vi "ADC Config Panel.vi"(8 "error in":errorcluster, 11 "adc session in":T2={"niScope"={"channel cfg"=[], "sessions"=[], "multi cards"=FALSE, "channels"=0, "type"=enum."n/a", "memory [B/chn]"=0, "ext. clock [Hz]"=0.0, "samples count"=0, "use streaming"=FALSE, "proc setup"={"packet size [smpl]"=0, "current timeout [s]"=0.0, "blk2blk timeout [s]"=0.0, "event time"=timestamp(0 s since 1904-01-01), "temp sampl T [s]"=0.0, "data queue"=refnum, "stop notifier"=refnum, "proc ref"=refnum}, "sample width [B]"=0, "ranges [V]"=[], "trigger setup"={"coupling"=1, "level [V]"=0.0, "slope"=0, "mode"=enum."Immediate", "pre-trigger [%]"=0.0}, "fs [Hz]"=0.0, "bitres [bit]"=0, "clock source"=enum."VAL_NO_SOURCE"}, "3458A"={"channels"=[], "sync unit"={"VISA"="", "type"=enum."Picotest U6200A"}, "awg unit"={"type"=enum."Agilent 331xxA to 332xxA", "VISA"="", "enable 10MHz ref"=FALSE, "cmi ckd2"={"VISA"="", "clock source"=enum."Auto", "manual ref clk"=FALSE, "ref clock [Hz]"=0.0, "div mode"=enum."Set divisor directly"}, "cmi sync v3"={"VISA"="", "baud rate [bd/s]"=115200, "source"=enum."Auto", "hv range"=enum."1kV", "fsrc is fixed"=FALSE, "fsrc [Hz]"=10000000.0, "freq integ [s]"=1.0, "freq filter"=5, "trig level"=enum."TTL 5V", "chn1 mode"=enum."Source divider", "chn1 level"=enum."Positive 5V", "chn2 mode"=enum."Source divider", "chn2 level"=enum."Positive 5V", "chn2 div"=1, "chn3 mode"=enum."Chn 1 Active", "chn3 level"=enum."Positive 5V", "chn1 div entry"=enum."Calculate nearest divisor from measured fx", "chn1 dev limit [%]"=1.0, "chn1 check dev"=FALSE}, "trigger"={"source"=enum."Immediate", "slope"=enum."POS", "coupling"=enum."DC", "level [V]"=0.0, "hysteresis [V]"=0.0, "pre-trigger [%]"=0.0}, "HMF2500 cfg"={"Baud Rate"=9600, "Parity"=0, "Data Bits"=8, "Flow Control"=4}}, "sync mode"=enum."MASTER-SLAVE, MASTER clocked by TIMER", "streaming mode"=FALSE, "idn mode"=enum."Auto", "sampling mode"=enum."DCV", "sample memory [B]"=0, "proc setup"={"channel id"=0, "packet size [smpl]"=0, "current timeout [s]"=0.0, "blk2blk timeout [s]"=0.0, "event time"=timestamp(0 s since 1904-01-01), "stop notifier"=refnum, "data queues"=[], "proc refs"=[], "bus semaphore"=refnum}, "sample size [B]"=0, "sample count"=0, "aux data"={"channel id"=0, "valid?"=[], "gain [V]"=[], "timestamp [s]"=[], "Ts [s]"=0.0, "abs timestamp"=timestamp(0 s since 1904-01-01), "t [deg C]"=[], "multiplex timestamp [s]"=-1.0, "only multiplex?"=FALSE, "multiplex smpl offset"=0, "overflow?"=FALSE}, "ranges [V]"=[], "aperture [s]"=0.0, "LEVEL trigger"={"edge"=enum."POS", "level [V]"=0.0, "coupling"=enum."DC"}, "trigger mode"=enum."AUTO", "measure temp.?"=FALSE, "disp mesages"=[], "shared bus?"=FALSE, "disable display?"=FALSE, "aper mode"=enum."Manual", "aper rules"=[], "multiplex"={"cycles"=0, "delay [s]"=0.0, "enabled"=FALSE, "overhead [s]"=1.0, "tot smpls"=0, "sub-rec"=0, "overhead [%]"=0.0, "emulated"=FALSE}, "F8588 lpf"=enum."Off", "F8588 pll"=enum."Off", "F8588 couple"=enum."DC, auto", "fs"={"freq mode"=enum."fs or Ts", "fs [Hz]"=0.0, "fref [Hz]"=0.0, "mul"=0.0, "div"=0.0}, "fs mode"=enum."fs or Ts"}, "dsdll"={"dsdll"={"dsdll path"=path "", "dsdll handle"=[], "output devices"=[], "capture devices"=[]}, "channels"=0, "device id"=0, "channel idns"=[], "proc setup"={"packet size [smpl]"=0, "current timeout [s]"=0.0, "blk2blk timeout [s]"=0.0, "event time"=timestamp(0 s since 1904-01-01), "data queue"=refnum, "stop notifier"=refnum, "proc ref"=refnum}, "samples count"=0, "fs [Hz]"=0.0}, "type"=enum."niScope", "channel idn str"=[], "aux instr idn str"=[], "modified?"=FALSE, "simadc"={"channels"=[], "range [V]"=0.0, "Ts step [s]"=0.0, "time [s]"=0.0, "fs [Hz]"=0.0, "count"=0, "smpl offset"=0, "set count"=0, "bit res"=0}, "force rst?"=FALSE, "exit mode"=enum."Immediate reset", "exit dly"=0.0, "exit tmr"=timestamp(0 s since 1904-01-01), "busy?"=FALSE, "accessed?"=FALSE, "multiplex"={"Type"=enum."Dummy", "gen com ssn"={"visa"="", "primary"=enum."None", "secondary"=enum."None", "channels"=[]}, "delay before [s]"=0.0, "delay post [s]"=0.0, "sequence"=[], "enabled"=FALSE, "ref timestamp [s]"=0.0, "idn string"="", "dev niScope"="", "niScope idx"=0, "QPMX ssn"={"visa"="", "switch mode"=enum."Switched by TWM", "sequence"=[], "timing delays"=[], "polarity"=enum."Positive", "ss delay (s)"=2.0, "internal timer (s)"=1.0, "Last loaded sequence file"=path "", "startup delay (s)"=2.0}, "VISA mux ssn"={"VISA"="", "paths"=[], "idn command"="", "serial cfg"={"Baud rate"=9600, "Data bits"=8, "Parity"=0, "Stop bits"=10, "Flow control"=0, "End Mode Read"=enum."None", "End Mode Write"=enum."None", "Term character"=0, "Term enable"=FALSE}}}, "keysight dso"={"VISA"="", "channels"=[], "bw limit [Hz]"=0.0, "resolution"=enum."Basic", "trig noise reject"=enum."Normal", "N"=0, "trigger config"={"trigger source"=enum."Immediate", "trigger slope"=enum."Negative", "level [V]"=0.0, "hysteresis [V]"=0.001, "pre-trig [%]"=50}, "fs [Hz]"=0.0, "timeout stop"=timestamp(0 s since 1904-01-01), "waiting for opc"=FALSE, "fetch offset [smpl]"=0, "abs timestamp"=timestamp(0 s since 1904-01-01), "ranges [V]"=[], "decimation"=0.0, "ext ref"=FALSE}, "cdaq"={"mclk [Hz]"=12800000.0, "ADC task"="", "mclk reference"="", "fs [Hz]"=50000.0, "queue adc cmd"=refnum, "queue adc data"=refnum, "adc proc ref"=refnum, "channels"=[], "last channels"=[], "timeout"=timestamp(0 s since 1904-01-01), "N"=1000, "mclk mode"=enum."Free running", "ext mclk source"=""}, "ignore overload"=FALSE} {"cdaq"."last channels"."Channel id" min=0 step=1; "cdaq"."channels"."Channel id" min=0 step=1; "keysight dso"."bw limit [Hz]" format="%#_6p"; "keysight dso"."channels"."Offset [V]" format="%#_6p"; "keysight dso"."channels"."Range [Vpk]" min=0.0 format="%#_6p"; "keysight dso"."channels"."Channel" min=1; "multiplex"."VISA mux ssn"."serial cfg"."Flow control" items=["None", "XON/XOFF", "CTS/RTS", "XON/XOFF + CTS/RTS", "DTR/DSR", "XON/XOFF + DTR/DSR"]; "multiplex"."VISA mux ssn"."serial cfg"."Stop bits" items=["1 bit"=10, "1.5 bits"=15, "2 bits"=20]; "multiplex"."VISA mux ssn"."serial cfg"."Parity" items=["None", "Odd", "Even", "Mark", "Space"]; "multiplex"."VISA mux ssn"."serial cfg"."Data bits" items=["5 bits"=5, "6 bits"=6, "7 bits"=7, "8 bits"=8]; "multiplex"."VISA mux ssn"."serial cfg"."Baud rate" items=["150 Bd"=150, "300 Bd"=300, "600 Bd"=600, "1200 Bd"=1200, "2400 Bd"=2400, "4800 Bd"=4800, "9600 Bd"=9600, "19.2 kBd"=19200, "38.4 kBd"=38400, "57.6 kBd"=57600, "115.2 kBd"=115200]; "multiplex"."QPMX ssn"."startup delay (s)" min=0.0 step=1.0; "multiplex"."QPMX ssn"."internal timer (s)" min=0.0 step=1.0; "multiplex"."QPMX ssn"."ss delay (s)" min=0.0 step=1.0; "multiplex"."QPMX ssn"."timing delays" min=1 max=255 step=1; "3458A"."awg unit"."HMF2500 cfg"."Flow Control" items=["None", "XON/XOFF", "RTS/CTS", "XON/XOFF & RTS/CTS", "DTR/DSR", "XON/XOFF & DTR/DSR"]; "3458A"."awg unit"."HMF2500 cfg"."Data Bits" items=["7"=7, "8"=8]; "3458A"."awg unit"."HMF2500 cfg"."Parity" items=["None", "Odd", "Even", "Mark", "Space"]; "3458A"."awg unit"."HMF2500 cfg"."Baud Rate" items=["300"=300, "600"=600, "1200"=1200, "2400"=2400, "4800"=4800, "9600"=9600, "19200"=19200]; "3458A"."awg unit"."cmi sync v3"."chn2 div" min=1 max=100000000 step=1; "3458A"."awg unit"."cmi sync v3"."fsrc [Hz]" format="%_8p"; "3458A"."channels"."Range [Vpk]" min=0.0; "niScope"."trigger setup"."pre-trigger [%]" format="%.2f"; "niScope"."trigger setup"."level [V]" format="%.2f"; "niScope"."trigger setup"."coupling" items=["AC"=0, "DC"=1, "HF Reject"=3, "LF Reject"=4, "AC Plus HF Reject"=1001]; "niScope"."channel cfg"."Range [Vpk]" min=0.0; "niScope"."channel cfg"."Channel" min=0}) -> (0 "error out":errorcluster, 3 "adc session out":T2={"niScope"={"channel cfg"=[], "sessions"=[], "multi cards"=FALSE, "channels"=0, "type"=enum."n/a", "memory [B/chn]"=0, "ext. clock [Hz]"=0.0, "samples count"=0, "use streaming"=FALSE, "proc setup"={"packet size [smpl]"=0, "current timeout [s]"=0.0, "blk2blk timeout [s]"=0.0, "event time"=timestamp(0 s since 1904-01-01), "temp sampl T [s]"=0.0, "data queue"=refnum, "stop notifier"=refnum, "proc ref"=refnum}, "sample width [B]"=0, "ranges [V]"=[], "trigger setup"={"coupling"=1, "level [V]"=0.0, "slope"=0, "mode"=enum."Immediate", "pre-trigger [%]"=0.0}, "fs [Hz]"=0.0, "bitres [bit]"=0, "clock source"=enum."VAL_NO_SOURCE"}, "3458A"={"channels"=[], "sync unit"={"VISA"="", "type"=enum."Picotest U6200A"}, "awg unit"={"type"=enum."Agilent 331xxA to 332xxA", "VISA"="", "enable 10MHz ref"=FALSE, "cmi ckd2"={"VISA"="", "clock source"=enum."Auto", "manual ref clk"=FALSE, "ref clock [Hz]"=0.0, "div mode"=enum."Set divisor directly"}, "cmi sync v3"={"VISA"="", "baud rate [bd/s]"=115200, "source"=enum."Auto", "hv range"=enum."1kV", "fsrc is fixed"=FALSE, "fsrc [Hz]"=10000000.0, "freq integ [s]"=1.0, "freq filter"=5, "trig level"=enum."TTL 5V", "chn1 mode"=enum."Source divider", "chn1 level"=enum."Positive 5V", "chn2 mode"=enum."Source divider", "chn2 level"=enum."Positive 5V", "chn2 div"=1, "chn3 mode"=enum."Chn 1 Active", "chn3 level"=enum."Positive 5V", "chn1 div entry"=enum."Calculate nearest divisor from measured fx", "chn1 dev limit [%]"=1.0, "chn1 check dev"=FALSE}, "trigger"={"source"=enum."Immediate", "slope"=enum."POS", "coupling"=enum."DC", "level [V]"=0.0, "hysteresis [V]"=0.0, "pre-trigger [%]"=0.0}, "HMF2500 cfg"={"Baud Rate"=9600, "Parity"=0, "Data Bits"=8, "Flow Control"=4}}, "sync mode"=enum."MASTER-SLAVE, MASTER clocked by TIMER", "streaming mode"=FALSE, "idn mode"=enum."Auto", "sampling mode"=enum."DCV", "sample memory [B]"=0, "proc setup"={"channel id"=0, "packet size [smpl]"=0, "current timeout [s]"=0.0, "blk2blk timeout [s]"=0.0, "event time"=timestamp(0 s since 1904-01-01), "stop notifier"=refnum, "data queues"=[], "proc refs"=[], "bus semaphore"=refnum}, "sample size [B]"=0, "sample count"=0, "aux data"={"channel id"=0, "valid?"=[], "gain [V]"=[], "timestamp [s]"=[], "Ts [s]"=0.0, "abs timestamp"=timestamp(0 s since 1904-01-01), "t [deg C]"=[], "multiplex timestamp [s]"=-1.0, "only multiplex?"=FALSE, "multiplex smpl offset"=0, "overflow?"=FALSE}, "ranges [V]"=[], "aperture [s]"=0.0, "LEVEL trigger"={"edge"=enum."POS", "level [V]"=0.0, "coupling"=enum."DC"}, "trigger mode"=enum."AUTO", "measure temp.?"=FALSE, "disp mesages"=[], "shared bus?"=FALSE, "disable display?"=FALSE, "aper mode"=enum."Manual", "aper rules"=[], "multiplex"={"cycles"=0, "delay [s]"=0.0, "enabled"=FALSE, "overhead [s]"=1.0, "tot smpls"=0, "sub-rec"=0, "overhead [%]"=0.0, "emulated"=FALSE}, "F8588 lpf"=enum."Off", "F8588 pll"=enum."Off", "F8588 couple"=enum."DC, auto", "fs"={"freq mode"=enum."fs or Ts", "fs [Hz]"=0.0, "fref [Hz]"=0.0, "mul"=0.0, "div"=0.0}, "fs mode"=enum."fs or Ts"}, "dsdll"={"dsdll"={"dsdll path"=path "", "dsdll handle"=[], "output devices"=[], "capture devices"=[]}, "channels"=0, "device id"=0, "channel idns"=[], "proc setup"={"packet size [smpl]"=0, "current timeout [s]"=0.0, "blk2blk timeout [s]"=0.0, "event time"=timestamp(0 s since 1904-01-01), "data queue"=refnum, "stop notifier"=refnum, "proc ref"=refnum}, "samples count"=0, "fs [Hz]"=0.0}, "type"=enum."niScope", "channel idn str"=[], "aux instr idn str"=[], "modified?"=FALSE, "simadc"={"channels"=[], "range [V]"=0.0, "Ts step [s]"=0.0, "time [s]"=0.0, "fs [Hz]"=0.0, "count"=0, "smpl offset"=0, "set count"=0, "bit res"=0}, "force rst?"=FALSE, "exit mode"=enum."Immediate reset", "exit dly"=0.0, "exit tmr"=timestamp(0 s since 1904-01-01), "busy?"=FALSE, "accessed?"=FALSE, "multiplex"={"Type"=enum."Dummy", "gen com ssn"={"visa"="", "primary"=enum."None", "secondary"=enum."None", "channels"=[]}, "delay before [s]"=0.0, "delay post [s]"=0.0, "sequence"=[], "enabled"=FALSE, "ref timestamp [s]"=0.0, "idn string"="", "dev niScope"="", "niScope idx"=0, "QPMX ssn"={"visa"="", "switch mode"=enum."Switched by TWM", "sequence"=[], "timing delays"=[], "polarity"=enum."Positive", "ss delay (s)"=2.0, "internal timer (s)"=1.0, "Last loaded sequence file"=path "", "startup delay (s)"=2.0}, "VISA mux ssn"={"VISA"="", "paths"=[], "idn command"="", "serial cfg"={"Baud rate"=9600, "Data bits"=8, "Parity"=0, "Stop bits"=10, "Flow control"=0, "End Mode Read"=enum."None", "End Mode Write"=enum."None", "Term character"=0, "Term enable"=FALSE}}}, "keysight dso"={"VISA"="", "channels"=[], "bw limit [Hz]"=0.0, "resolution"=enum."Basic", "trig noise reject"=enum."Normal", "N"=0, "trigger config"={"trigger source"=enum."Immediate", "trigger slope"=enum."Negative", "level [V]"=0.0, "hysteresis [V]"=0.001, "pre-trig [%]"=50}, "fs [Hz]"=0.0, "timeout stop"=timestamp(0 s since 1904-01-01), "waiting for opc"=FALSE, "fetch offset [smpl]"=0, "abs timestamp"=timestamp(0 s since 1904-01-01), "ranges [V]"=[], "decimation"=0.0, "ext ref"=FALSE}, "cdaq"={"mclk [Hz]"=12800000.0, "ADC task"="", "mclk reference"="", "fs [Hz]"=50000.0, "queue adc cmd"=refnum, "queue adc data"=refnum, "adc proc ref"=refnum, "channels"=[], "last channels"=[], "timeout"=timestamp(0 s since 1904-01-01), "N"=1000, "mclk mode"=enum."Free running", "ext mclk source"=""}, "ignore overload"=FALSE} {"cdaq"."last channels"."Channel id" min=0 step=1; "cdaq"."channels"."Channel id" min=0 step=1; "keysight dso"."bw limit [Hz]" format="%#_6p"; "keysight dso"."channels"."Offset [V]" format="%#_6p"; "keysight dso"."channels"."Range [Vpk]" min=0.0 format="%#_6p"; "keysight dso"."channels"."Channel" min=1; "multiplex"."VISA mux ssn"."serial cfg"."Flow control" items=["None", "XON/XOFF", "CTS/RTS", "XON/XOFF + CTS/RTS", "DTR/DSR", "XON/XOFF + DTR/DSR"]; "multiplex"."VISA mux ssn"."serial cfg"."Stop bits" items=["1 bit"=10, "1.5 bits"=15, "2 bits"=20]; "multiplex"."VISA mux ssn"."serial cfg"."Parity" items=["None", "Odd", "Even", "Mark", "Space"]; "multiplex"."VISA mux ssn"."serial cfg"."Data bits" items=["5 bits"=5, "6 bits"=6, "7 bits"=7, "8 bits"=8]; "multiplex"."VISA mux ssn"."serial cfg"."Baud rate" items=["150 Bd"=150, "300 Bd"=300, "600 Bd"=600, "1200 Bd"=1200, "2400 Bd"=2400, "4800 Bd"=4800, "9600 Bd"=9600, "19.2 kBd"=19200, "38.4 kBd"=38400, "57.6 kBd"=57600, "115.2 kBd"=115200]; "multiplex"."QPMX ssn"."startup delay (s)" min=0.0 step=1.0; "multiplex"."QPMX ssn"."internal timer (s)" min=0.0 step=1.0; "multiplex"."QPMX ssn"."ss delay (s)" min=0.0 step=1.0; "multiplex"."QPMX ssn"."timing delays" min=1 max=255 step=1; "3458A"."awg unit"."HMF2500 cfg"."Flow Control" items=["None", "XON/XOFF", "RTS/CTS", "XON/XOFF & RTS/CTS", "DTR/DSR", "XON/XOFF & DTR/DSR"]; "3458A"."awg unit"."HMF2500 cfg"."Data Bits" items=["7"=7, "8"=8]; "3458A"."awg unit"."HMF2500 cfg"."Parity" items=["None", "Odd", "Even", "Mark", "Space"]; "3458A"."awg unit"."HMF2500 cfg"."Baud Rate" items=["300"=300, "600"=600, "1200"=1200, "2400"=2400, "4800"=4800, "9600"=9600, "19200"=19200]; "3458A"."awg unit"."cmi sync v3"."chn2 div" min=1 max=100000000 step=1; "3458A"."awg unit"."cmi sync v3"."fsrc [Hz]" format="%_8p"; "3458A"."channels"."Range [Vpk]" min=0.0; "niScope"."trigger setup"."pre-trigger [%]" format="%.2f"; "niScope"."trigger setup"."level [V]" format="%.2f"; "niScope"."trigger setup"."coupling" items=["AC"=0, "DC"=1, "HF Reject"=3, "LF Reject"=4, "AC Plus HF Reject"=1001]; "niScope"."channel cfg"."Range [Vpk]" min=0.0; "niScope"."channel cfg"."Channel" min=0})   [LabVIEW 2020]
doc: "Configuration panel for digitizer."
uses:
  drivers/niScope/niScope Virtual Channel Config.ctl
  drivers/niScope/niScope Virtual Channel Mode.ctl
  drivers/niScope/niScope Virtual Channel Input Z.ctl
  drivers/niScope/niScope Virtual Channel Coupling.ctl
  ADC Type.ctl
  drivers/DMM/3458A Virtual Channel Config.ctl
  drivers/AWG/AWG Type.ctl
  drivers/DMM/3458A Idn Mode.ctl
  drivers/Counter/Counter Type.ctl
  drivers/DMM/3458A Digitizing Low Levels/Configure/Sampling Mode.ctl
  drivers/DMM/3458A Sync Mode.ctl
  ADC Session.ctl
  drivers/niScope/niScope Session.ctl
  drivers/niScope/niScope Type.ctl
  drivers/niScope/niScope Digitizing Process Options.ctl
  drivers/niScope/niScope Data Packet.ctl
  drivers/niScope/niScope Trigger Setup.ctl
  <instrlib>/niScope/Controls/niScope trigger coupling.ctl
  <instrlib>/niScope/Controls/niScope trigger slope.ctl
  drivers/niScope/niScope Reference Clock.ctl
  drivers/DMM/3458A Digitizer Session.ctl
  drivers/Counter/Counter Session.ctl
  drivers/AWG/AWG Session.ctl
  drivers/AWG/CMI Clock Divider v2/CMI ckd2 Session.ctl
  drivers/AWG/CMI Clock Divider v2/CMI ckd2 Source Mode.ctl
  drivers/AWG/CMI Clock Divider v2/CMI ckd2 Divisor Mode.ctl
  drivers/AWG/CMI Sync V3/CMI Sync V3 session.ctl
  drivers/AWG/CMI Sync V3/Configure/CMI Sync V3 Reference Clock Source.ctl
  drivers/AWG/CMI Sync V3/Configure/CMI Sync V3 HV input Range.ctl
  drivers/AWG/CMI Sync V3/Configure/CMI Sync V3 Trigger Input Level.ctl
  drivers/AWG/CMI Sync V3/Configure/CMI Sync V3 Channel 1 Mode.ctl
  drivers/AWG/CMI Sync V3/Configure/CMI Sync V3 Channel Output Levels.ctl
  drivers/AWG/CMI Sync V3/Configure/CMI Sync V3 Channel 2 Mode.ctl
  drivers/AWG/CMI Sync V3/Configure/CMI Sync V3 Channel 3 Mode.ctl
  drivers/AWG/CMI Sync V3/Configure/CMI Sync V3 Channel 1 Divisor Entry Mode.ctl
  ADC Trig Config.ctl
  ADC Trig Mode Source.ctl
  ADC Trig Slope.ctl
  ADC Trig Coupling.ctl
  drivers/AWG/RaS HMF2500/HMF2500 Config.ctl
  drivers/DMM/3458A Digitizing Process Options.ctl
  drivers/DMM/3458A Data Packet.ctl
  drivers/DMM/3458A Aux Record Data.ctl
  drivers/DMM/3458A Digitizing Low Levels/Configure/Level Setup.ctl
  drivers/DMM/3458A Digitizing Low Levels/Configure/First Sample Trigger.ctl
  drivers/DMM/3458A Aperture Selection Mode.ctl
  drivers/DMM/3458A Multiplexing Config.ctl
  drivers/Fluke 8588A/F8588A Low Pass Filter.ctl
  drivers/Fluke 8588A/F8588A Phase Lock.ctl
  drivers/Fluke 8588A/F8588A Coupling.ctl
  drivers/DMM/3458A Sampling Rate.ctl
  drivers/AWG/AWG Clock Setup Mode.ctl
  drivers/DMM/3458A Sample Rate Mode.ctl
  drivers/dsdll/DSDLL Session.ctl
  drivers/dsdll/dsdll/dsdll_instance.ctl
  drivers/dsdll/dsdll/dsdll_device_record.ctl
  drivers/dsdll/DSDLL Process Config.ctl
  drivers/dsdll/DSDLL Data Packet.ctl
  drivers/simulated_adc/SimAdc Config.ctl
  drivers/simulated_adc/SimAdc Channel Cfg.ctl
  ADC On Close Action.ctl
  Multiplexer/MPX Session.ctl
  Multiplexer/MPX Type.ctl
  drivers/Multiplexers/Generic COM/GCOMM Session.ctl
  drivers/Multiplexers/Generic COM/GCOMM Signal.ctl
  drivers/Multiplexers/Generic COM/GCOMM Virtual Channel.ctl
  drivers/Multiplexers/Generic COM/GCOMM Logic State.ctl
  drivers/Multiplexers/Generic COM/QPMX Session.ctl
  drivers/Multiplexers/QPMX/QPMX switch mode.ctl
  drivers/Multiplexers/QPMX/QPMX polarity.ctl
  drivers/Multiplexers/Generic VISA commands/GVISA Mux Session.ctl
  drivers/Multiplexers/Generic VISA commands/GVISA Mux Path Entry.ctl
  drivers/Multiplexers/Generic VISA commands/met_serial_setup.ctl
  drivers/Agilent DSO 90000/Virtual Digitizer/KeDSO session.ctl
  drivers/Agilent DSO 90000/Virtual Digitizer/KeDSO Virtual Channel.ctl
  drivers/Agilent DSO 90000/Virtual Digitizer/KeDSO High Resolution Mode.ctl
  drivers/Agilent DSO 90000/Virtual Digitizer/KeDSO Trigger Setup.ctl
  drivers/Agilent DSO 90000/Virtual Digitizer/KeDSO Trigger Source.ctl
  drivers/cdaq/cDAQ Session.ctl
  drivers/cdaq/low_level_old/cdaq_anal_adc_command.ctl
  drivers/cdaq/low_level_old/cdaq_anal_adc_data.ctl
  drivers/cdaq/cDAQ Virtual Channel.ctl
  drivers/cdaq/cDAQ Master Clock Mode.ctl
  varilib/SGUI Assign References Mode.ctl
  varilib/SGUI Assign Multiple Strings With Tags By Label.vi
  drivers/AWG/AWG.lvlib
  varilib/varilib.lvlib
  drivers/DMM/3458A Virtual Digitizer.lvlib
  drivers/AWG/CMI Sync V3/CMI Sync Unit V3.lvlib
  drivers/niScope/niScope Virtual Digitizer.lvlib
  drivers/DMM/3458A Digitizing Low Levels/3458A Digitizing Low Levels.lvlib
  drivers/Counter/Counter.lvlib
  drivers/dsdll/DSDLL Virtual Digitizer.lvlib
  drivers/dsdll/dsdll/dsdll.lvlib
panel:
  in  "help":bool caption="Help"
  in  "btn default":bool
  in  "tc on exit 2":enum32{"Page 1"}(tab)
  in  "mpx on":bool caption="Enable multiplexer mode"
  in  "btn mpx":bool
  in  "tc on exit":enum32{"Page 1"}(tab)
  in  "ignore ovrld":bool caption="Ignore channel overload"
  in  "exit delay":dbl=30.0 caption="Delay [s]"
  in  "exit mode":T1 caption="On device close"
  in  "force rst":bool caption="Force reset on open"
  in  "btn selfcal":bool
  in  "tc idn":enum32{"Page 1"}(tab)
  out "adcstr":string caption="Identification/Status:"
  in  "btn test":bool
  in  "btn cancel":bool
  in  "btn ok":bool
  in  "tc cfg":T80(tab)
  in  "niSc clock mode":T13 caption="External clock mode"
  in  "btn rem last niScope":bool
  in  "niSc streaming":bool caption="Use streaming mode"
  in  "niSc ext clock":dbl caption="External clock [Hz]" format="%#_6p"
  in  "btn clr niScope":bool
  in  "niSc channels":T4[](array[typedef]) caption="ADC Channels" {"Range [Vpk]" min=0.0; "Channel" min=0}
  in  "btn dmm calstr":bool
  in  "dmm couple":T49=enum."DC, auto" caption="Fluke 8588A coupling"
  in  "dmm 8588 pll":T48 caption="Fluke 8588A phase lock"
  in  "dmm lpf":T47 caption="Fluke 8588A Low Pass"
  in  "DMM Channels":T15[](array[typedef]) {"Range [Vpk]" min=0.0}
  in  "dmm aper mode":T45 caption="Aperture selection mode"
  in  "dmm aper rules":string[][](table) caption="Aperture selection rules (popup menu)"
  in  "dmm disable disp":bool caption="Disable display"
  in  "btn rem last dmm":bool
  in  "dmm meas t":bool caption="Measure temperature"
  in  "dmm stream":bool caption="Use streaming mode"
  in  "dmm sync mode":T37 caption="Synchronization mode"
  in  "counter VISA":refnum<visa-resource-name> caption="Counter VISA"
  in  "AWG VISA":refnum<visa-resource-name>
  in  "counter type":T17 caption="Counter type"
  in  "AWG ext ref":bool caption="Use external\n10 MHz for AWG"
  in  "AWG type":T19
  in  "btn clr dmm":bool
  in  "dmm idn mode":T38 caption="DMM descriptor mode"
  in  "dmm smpl mode":T39 caption="DMM digitizing mode"
  in  "btn cfg AWG":bool
  in  "dmm fs mode":T52 caption="Alternative sampling rate mode"
  in  "btn dsdll enum":bool
  in  "dsdll channels":i32=1 caption="Channels count (1 or 2)" min=1 max=2 step=1
  in  "dsdll capt devs":u16(ring) caption="Capture devices"
  in  "keDSO ext ref":bool caption="Use external clock reference"
  in  "keDSO high res":T74 caption="Bit resolution"
  in  "keDSO visa":refnum<visa-resource-name> caption="Scope VISA address"
  in  "keDSO trg noise rj":enum16{"Normal", "High Sensitivity"}(ring) caption="Trigger noise reject"
  in  "keDSO bw limit":dbl=-1.0 caption="Bandwidth limit [Hz]" format="%#_6p"
  in  "keDSO channels":T73[](array[typedef]) caption="ADC Channels" {"Offset [V]" format="%#_6p"; "Range [Vpk]" min=0.0 format="%#_6p"; "Channel" min=1}
  in  "btn rem last cdaq":bool
  in  "btn clr cdaq":bool
  out "cDAQ proc running":bool caption="Digitizing process is running"
  out "cDAQ mckl ref":string caption="Selected MasterClock reference name (for exporting to another device running in another application)"
  in  "cDAQ fs [Hz]":dbl caption="Fixed sampling rate [Sa/s]" format="%#_6p"
  in  "cDAQ chns":T78[](array[typedef]) caption="ADC channels" {"Channel id" min=0 step=1}
  in  "cDAQ ext mclk src":tag caption="External master clock source"
  in  "cDAQ mclk mode":T79 caption="Digitizer master clock mode"
  in  "cDAQ mclk [Hz]":dbl caption="External master clock frequency [Hz]" format="%#_8p"
  in  "simadc bitres":i32=16 caption="ADC resolution [bit]"
  in  "Range [V]":dbl
  in  "Sampling period step [s]":dbl
  in  "btn sim clr":bool caption="Clear List"
  in  "simadc chn cfg":T59[](array[typedef]) caption="Channel signal definitions"
  in  "tc type":enum32{"Page 1"}(tab)
  out "Description":string
  in  "Digitizer type":T57
  # "- Use 0 for internal clock"
  # "- use '-1' to disable BW limit"
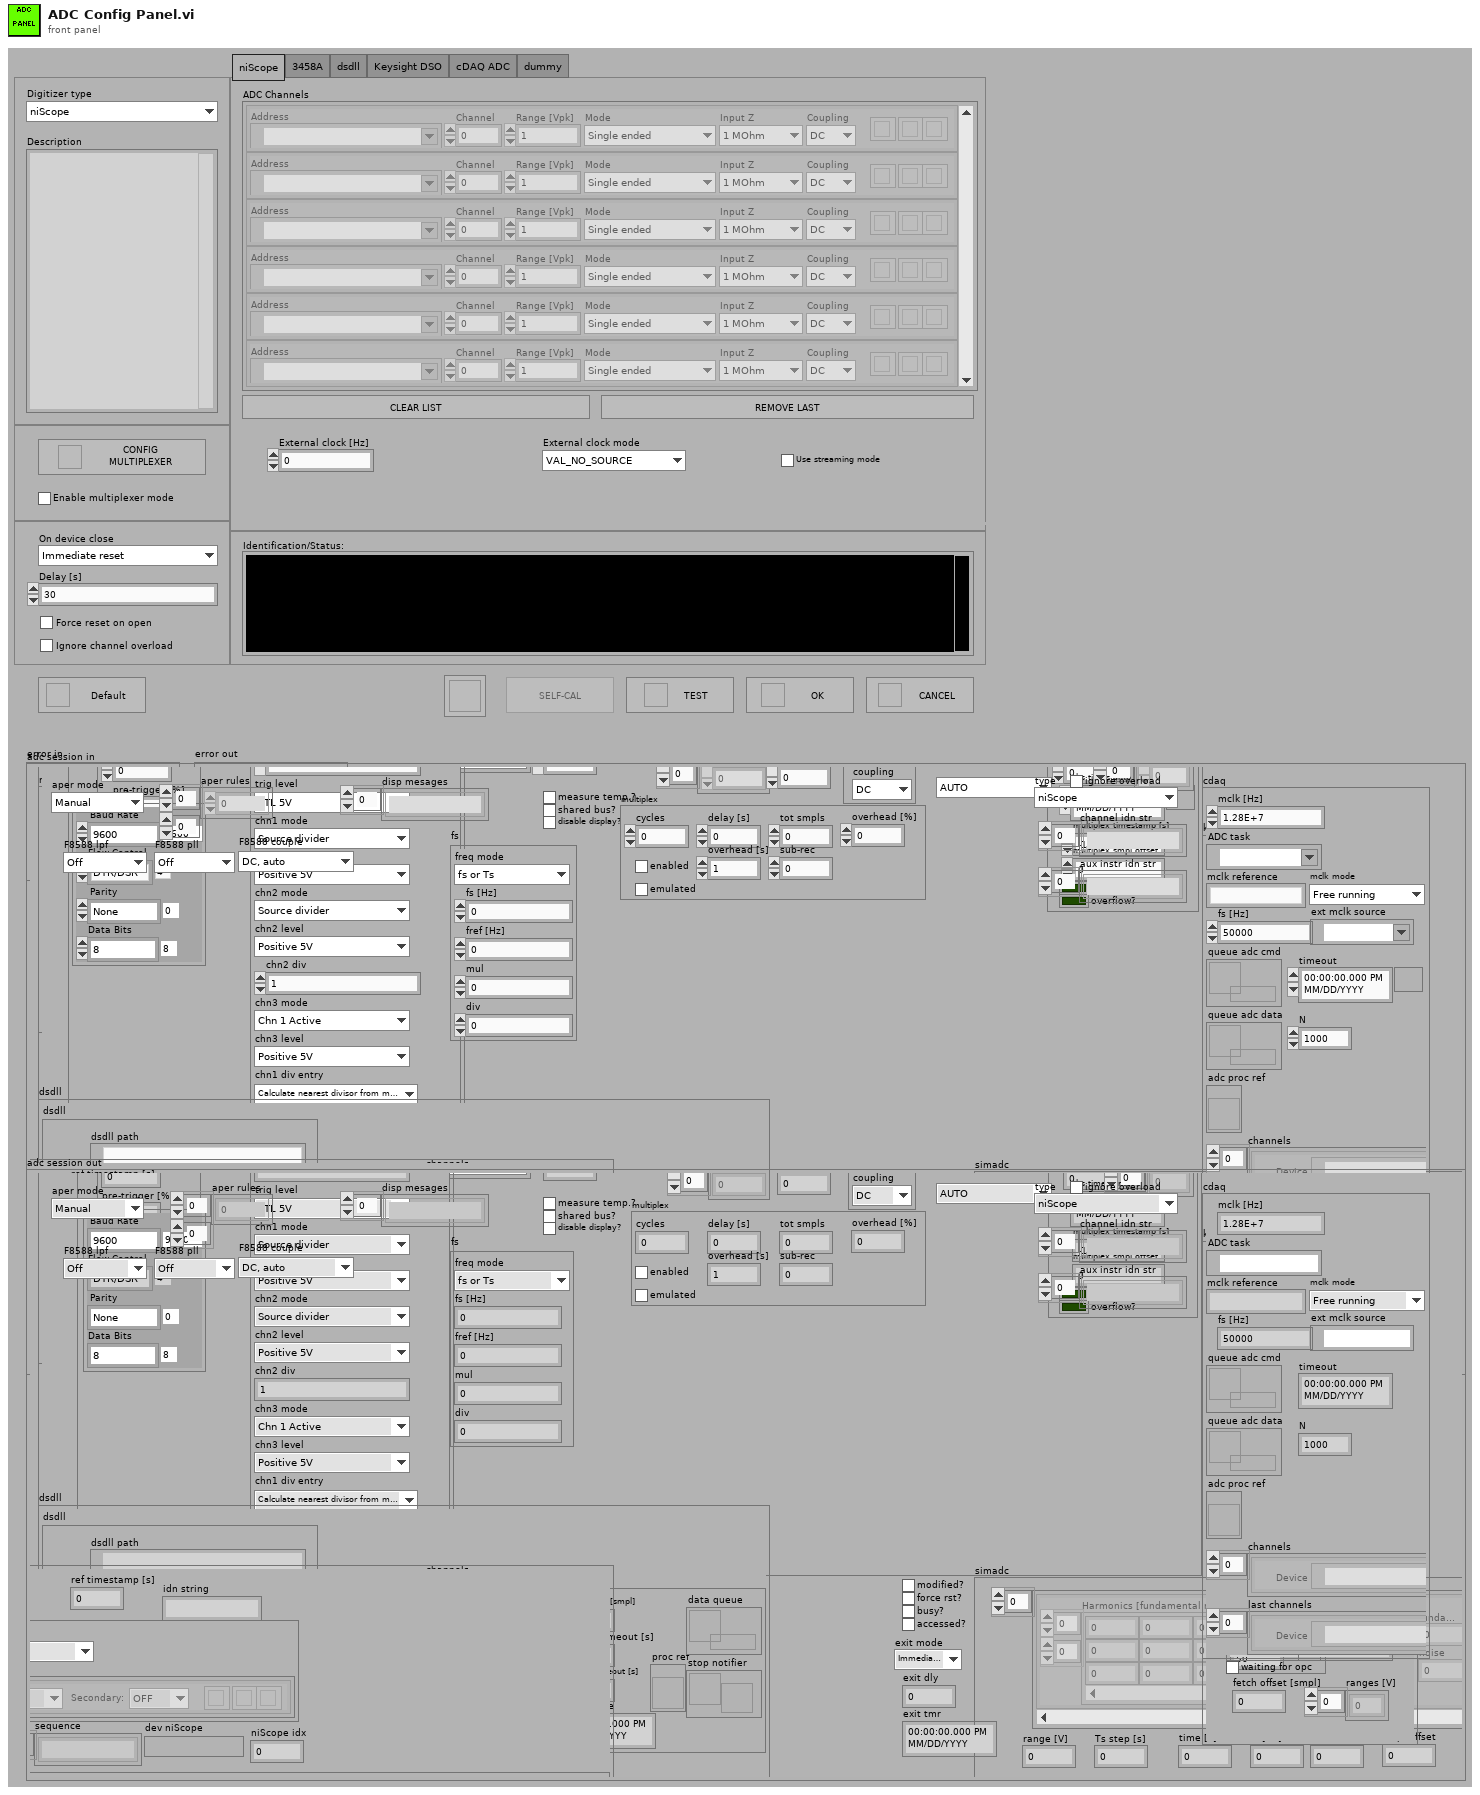
[diagram p1: front panel]
types:
  T1 = typedef "ADC On Close Action.ctl" = enum16{"Immediate reset", "Delayed reset"}
  T2 = typedef "ADC Session.ctl" = cluster{"niScope":T3, "3458A":T14, "dsdll":T53, "type":T57, "channel idn str":string[], "aux instr idn str":string[], "modified?":bool, "simadc":T58, "force rst?":bool, "exit mode":T1, "exit dly":dbl, "exit tmr":timestamp, "busy?":bool, "accessed?":bool, "multiplex":T60, "keysight dso":T72, "cdaq":T77, "ignore overload":bool}
  T3 = typedef "niScope Virtual Digitizer.lvlib/niScope Session.ctl" = cluster{"channel cfg":T4[], "sessions":refnum<k20>[], "multi cards":bool, "channels":i32, "type":T8, "memory [B/chn]":i32, "ext. clock [Hz]":dbl, "samples count":i64, "use streaming":bool, "proc setup":T9, "sample width [B]":i32, "ranges [V]":dbl[], "trigger setup":T10, "fs [Hz]":dbl, "bitres [bit]":i32, "clock source":T13}
  T4 = typedef "niScope Virtual Digitizer.lvlib/niScope Virtual Channel Config.ctl" = cluster{"Address":refnum<k15>, "Channel":i32, "Mode":T5, "Input Z":T6, "Coupling":T7, "Range [Vpk]":dbl, "btn clr":bool, "btn up":bool, "btn down":bool}
  T5 = typedef "niScope Virtual Digitizer.lvlib/niScope Virtual Channel Mode.ctl" = enum16{"Single ended", "Unbal. differential", "Differential"}
  T6 = typedef "niScope Virtual Digitizer.lvlib/niScope Virtual Channel Input Z.ctl" = enum16{"1 MOhm", "50 Ohm"}
  T7 = typedef "niScope Virtual Digitizer.lvlib/niScope Virtual Channel Coupling.ctl" = enum16{"AC", "DC", "GND"}
  T8 = typedef "niScope Virtual Digitizer.lvlib/niScope Type.ctl" = enum16{"n/a", "5922"}
  T9 = typedef "niScope Virtual Digitizer.lvlib/niScope Digitizing Process Options.ctl" = cluster{"packet size [smpl]":i64, "current timeout [s]":dbl, "blk2blk timeout [s]":dbl, "event time":timestamp, "temp sampl T [s]":dbl, "data queue":refnum<queue>, "stop notifier":refnum<notifier>, "proc ref":refnum<vi>}
  T10 = typedef "niScope Virtual Digitizer.lvlib/niScope Trigger Setup.ctl" = cluster{"coupling":T11, "level [V]":dbl, "slope":T12, "mode":enum16{"Immediate", "External", "Level"}, "pre-trigger [%]":dbl}
  T11 = typedef "niScope trigger coupling.ctl" = u16
  T12 = typedef "niScope trigger slope.ctl" = i32
  T13 = typedef "niScope Virtual Digitizer.lvlib/niScope Reference Clock.ctl" = enum16{"VAL_NO_SOURCE", "VAL_CLK_IN", "VAL_PXI_CLOCK", "VAL_EXTERNAL"}
  T14 = typedef "3458A Virtual Digitizer.lvlib/3458A Digitizer Session.ctl" = cluster{"channels":T15[], "sync unit":T16, "awg unit":T18, "sync mode":T37, "streaming mode":bool, "idn mode":T38, "sampling mode":T39, "sample memory [B]":i32, "proc setup":T40, "sample size [B]":i32, "sample count":i32, "aux data":T42, "ranges [V]":dbl[], "aperture [s]":dbl, "LEVEL trigger":T43, "trigger mode":T44, "measure temp.?":bool, "disp mesages":string[], "shared bus?":bool, "disable display?":bool, "aper mode":T45, "aper rules":dbl[][], "multiplex":T46, "F8588 lpf":T47, "F8588 pll":T48, "F8588 couple":T49, "fs":T50, "fs mode":T52}
  T15 = typedef "3458A Virtual Digitizer.lvlib/3458A Virtual Channel Config.ctl" = cluster{"VISA":refnum<visa-resource-name>, "Range [Vpk]":dbl, "btn clr":bool, "btn up":bool, "btn down":bool, "F8588":bool, "F8588 guard":bool}
  T16 = typedef "Counter.lvlib/Counter Session.ctl" = cluster{"VISA":refnum<visa-resource-name>, "type":T17}
  T17 = typedef "Counter.lvlib/Counter Type.ctl" = enum16{"Picotest U6200A", "dummy"}
  T18 = typedef "AWG.lvlib/AWG Session.ctl" = cluster{"type":T19, "VISA":refnum<visa-resource-name>, "enable 10MHz ref":bool, "cmi ckd2":T20, "cmi sync v3":T23, "trigger":T32, "HMF2500 cfg":T36}
  T19 = typedef "AWG.lvlib/AWG Type.ctl" = enum16{"Agilent 331xxA to 332xxA", "Agilent 335xxA to 336xxA", "Tektronix AFG3101C", "R&S HMF25xx", "CMI Clock Divider v2", "CMI Sync Unit V3", "dummy"}
  T20 = typedef "AWG.lvlib/CMI ckd2 Session.ctl" = cluster{"VISA":refnum<visa-resource-name>, "clock source":T21, "manual ref clk":bool, "ref clock [Hz]":dbl, "div mode":T22}
  T21 = typedef "AWG.lvlib/CMI ckd2 Source Mode.ctl" = enum16{"Auto", "LF clock", "HF clock", "Internal"}
  T22 = typedef "AWG.lvlib/CMI ckd2 Divisor Mode.ctl" = enum16{"Set divisor directly", "Set divisor by frequency"}
  T23 = typedef "AWG.lvlib/CMI Sync Unit V3.lvlib/CMI Sync V3 session.ctl" = cluster{"VISA":refnum<visa-resource-name>, "baud rate [bd/s]":i32, "source":T24, "hv range":T25, "fsrc is fixed":bool, "fsrc [Hz]":dbl, "freq integ [s]":dbl, "freq filter":i32, "trig level":T26, "chn1 mode":T27, "chn1 level":T28, "chn2 mode":T29, "chn2 level":T28, "chn2 div":i32, "chn3 mode":T30, "chn3 level":T28, "chn1 div entry":T31, "chn1 dev limit [%]":dbl, "chn1 check dev":bool}
  T24 = typedef "AWG.lvlib/CMI Sync Unit V3.lvlib/CMI Sync V3 Reference Clock Source.ctl" = enum16{"Auto", "Internal", "Logic", "Sine", "HV"}
  T25 = typedef "AWG.lvlib/CMI Sync Unit V3.lvlib/CMI Sync V3 HV input Range.ctl" = enum16{"10V", "60V", "250V", "1kV"}
  T26 = typedef "AWG.lvlib/CMI Sync Unit V3.lvlib/CMI Sync V3 Trigger Input Level.ctl" = enum16{"LVCMOS 3V3", "TTL 5V"}
  T27 = typedef "AWG.lvlib/CMI Sync Unit V3.lvlib/CMI Sync V3 Channel 1 Mode.ctl" = enum16{"Source divider", "DDS absolute", "DDS ratio", "DDS ratio M/N"}
  T28 = typedef "AWG.lvlib/CMI Sync Unit V3.lvlib/CMI Sync V3 Channel Output Levels.ctl" = enum16{"Positive 3V3", "Negative 3V3", "Positive 5V", "Negative 5V"}
  T29 = typedef "AWG.lvlib/CMI Sync Unit V3.lvlib/CMI Sync V3 Channel 2 Mode.ctl" = enum16{"Source divider", "Chn 1 divide"}
  T30 = typedef "AWG.lvlib/CMI Sync Unit V3.lvlib/CMI Sync V3 Channel 3 Mode.ctl" = enum16{"Chn 1 Active", "Chn 2 Active", "Chn 1 Trigger", "Chn 2 Trigger", "Gate", "PPS", "10MHz"}
  T31 = typedef "AWG.lvlib/CMI Sync Unit V3.lvlib/CMI Sync V3 Channel 1 Divisor Entry Mode.ctl" = enum16{"Set divisor directly", "Calculate nearest divisor from measured fx"}
  T32 = typedef "ADC Trig Config.ctl" = cluster{"source":T33, "slope":T34, "coupling":T35, "level [V]":dbl, "hysteresis [V]":dbl, "pre-trigger [%]":dbl}
  T33 = typedef "ADC Trig Mode Source.ctl" = enum16{"Immediate", "External", "Level"}
  T34 = typedef "ADC Trig Slope.ctl" = enum16{"POS", "NEG"}
  T35 = typedef "ADC Trig Coupling.ctl" = enum16{"DC", "AC"}
  T36 = typedef "AWG.lvlib/HMF2500 Config.ctl" = cluster{"Baud Rate":u32, "Parity":u16, "Data Bits":u16, "Flow Control":u16}
  T37 = typedef "3458A Virtual Digitizer.lvlib/3458A Sync Mode.ctl" = enum16{"MASTER-SLAVE, MASTER clocked by TIMER", "MASTER-SLAVE, MASTER clocked by AWG", "ALL clocked by AWG", "MASTER-SLAVE, ALL clocked by TIMER", "ALL clocked by AWG with DFLL"}
  T38 = typedef "3458A Virtual Digitizer.lvlib/3458A Idn Mode.ctl" = enum16{"Auto", "Sequential (chn A, chn B, ...)", "From calibration string"}
  T39 = typedef "3458A Virtual Digitizer.lvlib/3458A Digitizing Low Levels.lvlib/Sampling Mode.ctl" = enum16{"DCV", "DSDC", "DSAC"}
  T40 = typedef "3458A Virtual Digitizer.lvlib/3458A Digitizing Process Options.ctl" = cluster{"channel id":i32, "packet size [smpl]":i32, "current timeout [s]":dbl, "blk2blk timeout [s]":dbl, "event time":timestamp, "stop notifier":refnum<notifier>, "data queues":refnum<queue>[], "proc refs":refnum<vi>[], "bus semaphore":T41}
  T41 = typedef "Semaphore RefNum" = refnum<k1>
  T42 = typedef "3458A Virtual Digitizer.lvlib/3458A Aux Record Data.ctl" = cluster{"channel id":i32, "valid?":bool[], "gain [V]":dbl[], "timestamp [s]":dbl[], "Ts [s]":dbl, "abs timestamp":timestamp, "t [deg C]":dbl[], "multiplex timestamp [s]":dbl, "only multiplex?":bool, "multiplex smpl offset":i64, "overflow?":bool}
  T43 = typedef "3458A Virtual Digitizer.lvlib/3458A Digitizing Low Levels.lvlib/Level Setup.ctl" = cluster{"edge":enum16{"POS", "NEG"}, "level [V]":dbl, "coupling":enum16{"DC", "AC"}}
  T44 = typedef "3458A Virtual Digitizer.lvlib/3458A Digitizing Low Levels.lvlib/First Sample Trigger.ctl" = enum16{"AUTO", "EXT", "SYN", "SGL", "HOLD", "LEVEL"}
  T45 = typedef "3458A Virtual Digitizer.lvlib/3458A Aperture Selection Mode.ctl" = enum16{"Manual", "Maximum", "Table"}
  T46 = typedef "3458A Virtual Digitizer.lvlib/3458A Multiplexing Config.ctl" = cluster{"cycles":i32, "delay [s]":dbl, "enabled":bool, "overhead [s]":dbl, "tot smpls":i64, "sub-rec":i32, "overhead [%]":dbl, "emulated":bool}
  T47 = typedef "F8588A Low Pass Filter.ctl" = enum16{"Off", "100 kHz", "3 MHz"}
  T48 = typedef "F8588A Phase Lock.ctl" = enum16{"Off", "1 MHz", "10 MHz"}
  T49 = typedef "F8588A Coupling.ctl" = enum16{"AC, 1 MOhm", "AC, 10 MOhm", "DC, 1 MOhm", "DC, 10 MOhm", "DC, auto"}
  T50 = typedef "3458A Virtual Digitizer.lvlib/3458A Sampling Rate.ctl" = cluster{"freq mode":T51, "fs [Hz]":dbl, "fref [Hz]":dbl, "mul":dbl, "div":dbl}
  T51 = typedef "AWG.lvlib/AWG Clock Setup Mode.ctl" = enum16{"fs or Ts", "fs or Ts with fref", "fref/N", "fref*M/N", "fref*Ratio"}
  T52 = typedef "3458A Sample Rate Mode.ctl" = enum16{"fs or Ts", "fs*M/N"}
  T53 = typedef "DSDLL Virtual Digitizer.lvlib/DSDLL Session.ctl" = cluster{"dsdll":T54, "channels":i32, "device id":i32, "channel idns":string[], "proc setup":T56, "samples count":i32, "fs [Hz]":dbl}
  T54 = typedef "dsdll.lvlib/dsdll_instance.ctl" = cluster{"dsdll path":path, "dsdll handle":u8[], "output devices":T55[], "capture devices":T55[]}
  T55 = typedef "dsdll.lvlib/dsdll_device_record.ctl" = cluster{"guid":u8[], "name":string}
  T56 = typedef "DSDLL Virtual Digitizer.lvlib/DSDLL Process Config.ctl" = cluster{"packet size [smpl]":i32, "current timeout [s]":dbl, "blk2blk timeout [s]":dbl, "event time":timestamp, "data queue":refnum<queue>, "stop notifier":refnum<notifier>, "proc ref":refnum<vi>}
  T57 = typedef "ADC Type.ctl" = enum16{"niScope", "3458A", "DirectSound DLL", "Keysight DSO", "cDAQ ADC", "dummy"}
  T58 = typedef "SimAdc Config.ctl" = cluster{"channels":T59[], "range [V]":dbl, "Ts step [s]":dbl, "time [s]":dbl, "fs [Hz]":dbl, "count":i64, "smpl offset":i64, "set count":i64, "bit res":i32}
  T59 = typedef "SimAdc Channel Cfg.ctl" = cluster{"harmonics":dbl[][], "btn clear":bool, "noise":dbl, "fundamental [Hz]":dbl}
  T60 = typedef "MPX Session.ctl" = cluster{"Type":T61, "gen com ssn":T62, "delay before [s]":dbl, "delay post [s]":dbl, "sequence":string[], "enabled":bool, "ref timestamp [s]":dbl, "idn string":string, "dev niScope":refnum<k15>, "niScope idx":i32, "QPMX ssn":T66, "VISA mux ssn":T69}
  T61 = typedef "MPX Type.ctl" = enum16{"Dummy", "Generic - COM port", "Generic - niScope PFI", "Generic - VISA commands", "QPMX"}
  T62 = typedef "GCOMM Session.ctl" = cluster{"visa":refnum<visa-resource-name>, "primary":T63, "secondary":T63, "channels":T64[]}
  T63 = typedef "GCOMM Signal.ctl" = enum16{"None", "DTR", "RTS"}
  T64 = typedef "GCOMM Virtual Channel.ctl" = cluster{"Primary:":T65, "Secondary:":T65, "btn clr":bool, "btn up":bool, "btn down":bool, "Tag:":string}
  T65 = typedef "GCOMM Logic State.ctl" = enum16{"OFF", "ON"}
  T66 = typedef "QPMX Session.ctl" = cluster{"visa":refnum<visa-resource-name>, "switch mode":T67, "sequence":bool[][], "timing delays":u32[], "polarity":T68, "ss delay (s)":dbl, "internal timer (s)":dbl, "Last loaded sequence file":path, "startup delay (s)":dbl}
  T67 = typedef "QPMX switch mode.ctl" = enum16{"Switched by TWM", "Switched by external clock", "Switched by internal clock"}
  T68 = typedef "QPMX polarity.ctl" = enum16{"Positive", "Negative"}
  T69 = typedef "GVISA Mux Session.ctl" = cluster{"VISA":refnum<visa-resource-name>, "paths":T70[], "idn command":string, "serial cfg":T71}
  T70 = typedef "GVISA Mux Path Entry.ctl" = cluster{"Tag:":string, "Command:":string, "btn clr":bool, "btn up":bool, "btn down":bool}
  T71 = typedef "met_serial_setup.ctl" = cluster{"Baud rate":i32, "Data bits":i32, "Parity":i32, "Stop bits":i32, "Flow control":i32, "End Mode Read":enum16{"None", "Last Bit", "TermChar"}, "End Mode Write":enum16{"None", "Last Bit", "TermChar"}, "Term character":u8, "Term enable":bool}
  T72 = typedef "KeDSO session.ctl" = cluster{"VISA":refnum<visa-resource-name>, "channels":T73[], "bw limit [Hz]":dbl, "resolution":T74, "trig noise reject":enum16{"Normal", "High Sensitivity"}, "N":i64, "trigger config":T75, "fs [Hz]":dbl, "timeout stop":timestamp, "waiting for opc":bool, "fetch offset [smpl]":i64, "abs timestamp":timestamp, "ranges [V]":dbl[], "decimation":dbl, "ext ref":bool}
  T73 = typedef "KeDSO Virtual Channel.ctl" = cluster{"Channel":i32, "Range [Vpk]":dbl, "btn clr":bool, "btn up":bool, "btn down":bool, "Offset [V]":dbl, "Coupling":enum16{"DC", "DC50", "AC", "LFR1"}, "bw limit enab":bool}
  T74 = typedef "KeDSO High Resolution Mode.ctl" = enum16{"Basic", "High-res AUTO", "Min. 9-bits", "Min. 10-bits", "Min. 11-bits", "Min. 12-bits", "Fixed 11-bits", "Fixed 12-bits", "Fixed 13-bits", "Fixed 14-bits", "Fixed 15-bits", "Fixed 16-bits"}
  T75 = typedef "KeDSO Trigger Setup.ctl" = cluster{"trigger source":T76, "trigger slope":enum16{"Negative", "Positive", "Either"}, "level [V]":dbl, "hysteresis [V]":dbl, "pre-trig [%]":i32}
  T76 = typedef "KeDSO Trigger Source.ctl" = enum16{"Immediate", "Level", "AUX"}
  T77 = typedef "cDAQ Session.ctl" = cluster{"mclk [Hz]":dbl, "ADC task":refnum<k21>, "mclk reference":string, "fs [Hz]":dbl, "queue adc cmd":refnum<queue>, "queue adc data":refnum<queue>, "adc proc ref":refnum<vi>, "channels":T78[], "last channels":T78[], "timeout":timestamp, "N":i32, "mclk mode":T79, "ext mclk source":tag}
  T78 = typedef "cDAQ Virtual Channel.ctl" = cluster{"Device":tag, "Channel id":i32, "btn clr":bool, "btn up":bool, "btn down":bool}
  T79 = typedef "cDAQ Master Clock Mode.ctl" = enum16{"Free running", "Export master clock", "Import master clock"}
  T80 = enum32{"niScope", "3458A", "dsdll", "Keysight DSO", "cDAQ ADC", "dummy"}
  T81 = typedef "varilib.lvlib/SGUI Assign References Mode.ctl" = enum16{"Add to stack", "Overwrite", "Release last", "Release ID"}
  T82 = typedef "ADC Capabilities.ctl" = cluster{"max samples count":i64, "max fs [Hz]":ext, "min fs [Hz]":ext, "Ts step [s]":ext, "max Ts [s]":ext, "min Ts [s]":ext, "allows streaming?":bool, "streaming on?":bool, "has level trig?":bool, "has ext trig?":bool, "has aperture?":bool, "aper min [s]":dbl, "aper max [s]":dbl, "channels count":i32, "has ranges?":bool, "has temperature?":bool, "has temperature log?":bool, "has selfcal?":bool, "fs step [Hz]":ext, "smpl rate step mode":T83, "no aper info":string, "no fs info":string, "has fs?":bool, "srate mode":T51, "auto aperture?":bool, "auto aperture [s]":ext, "user fs mode option?":bool, "has pre-trigger?":bool, "has trigger hyst?":bool}
  T83 = typedef "ADC Sampling Rate Step Mode.ctl" = enum16{"const period", "const frequency"}
  T84 = typedef "ADC Status.ctl" = cluster{"cDAQ":T85}
  T85 = typedef "cDAQ Status.ctl" = cluster{"mclk [Hz]":dbl, "mckl reference":string, "digitizing process running":bool}
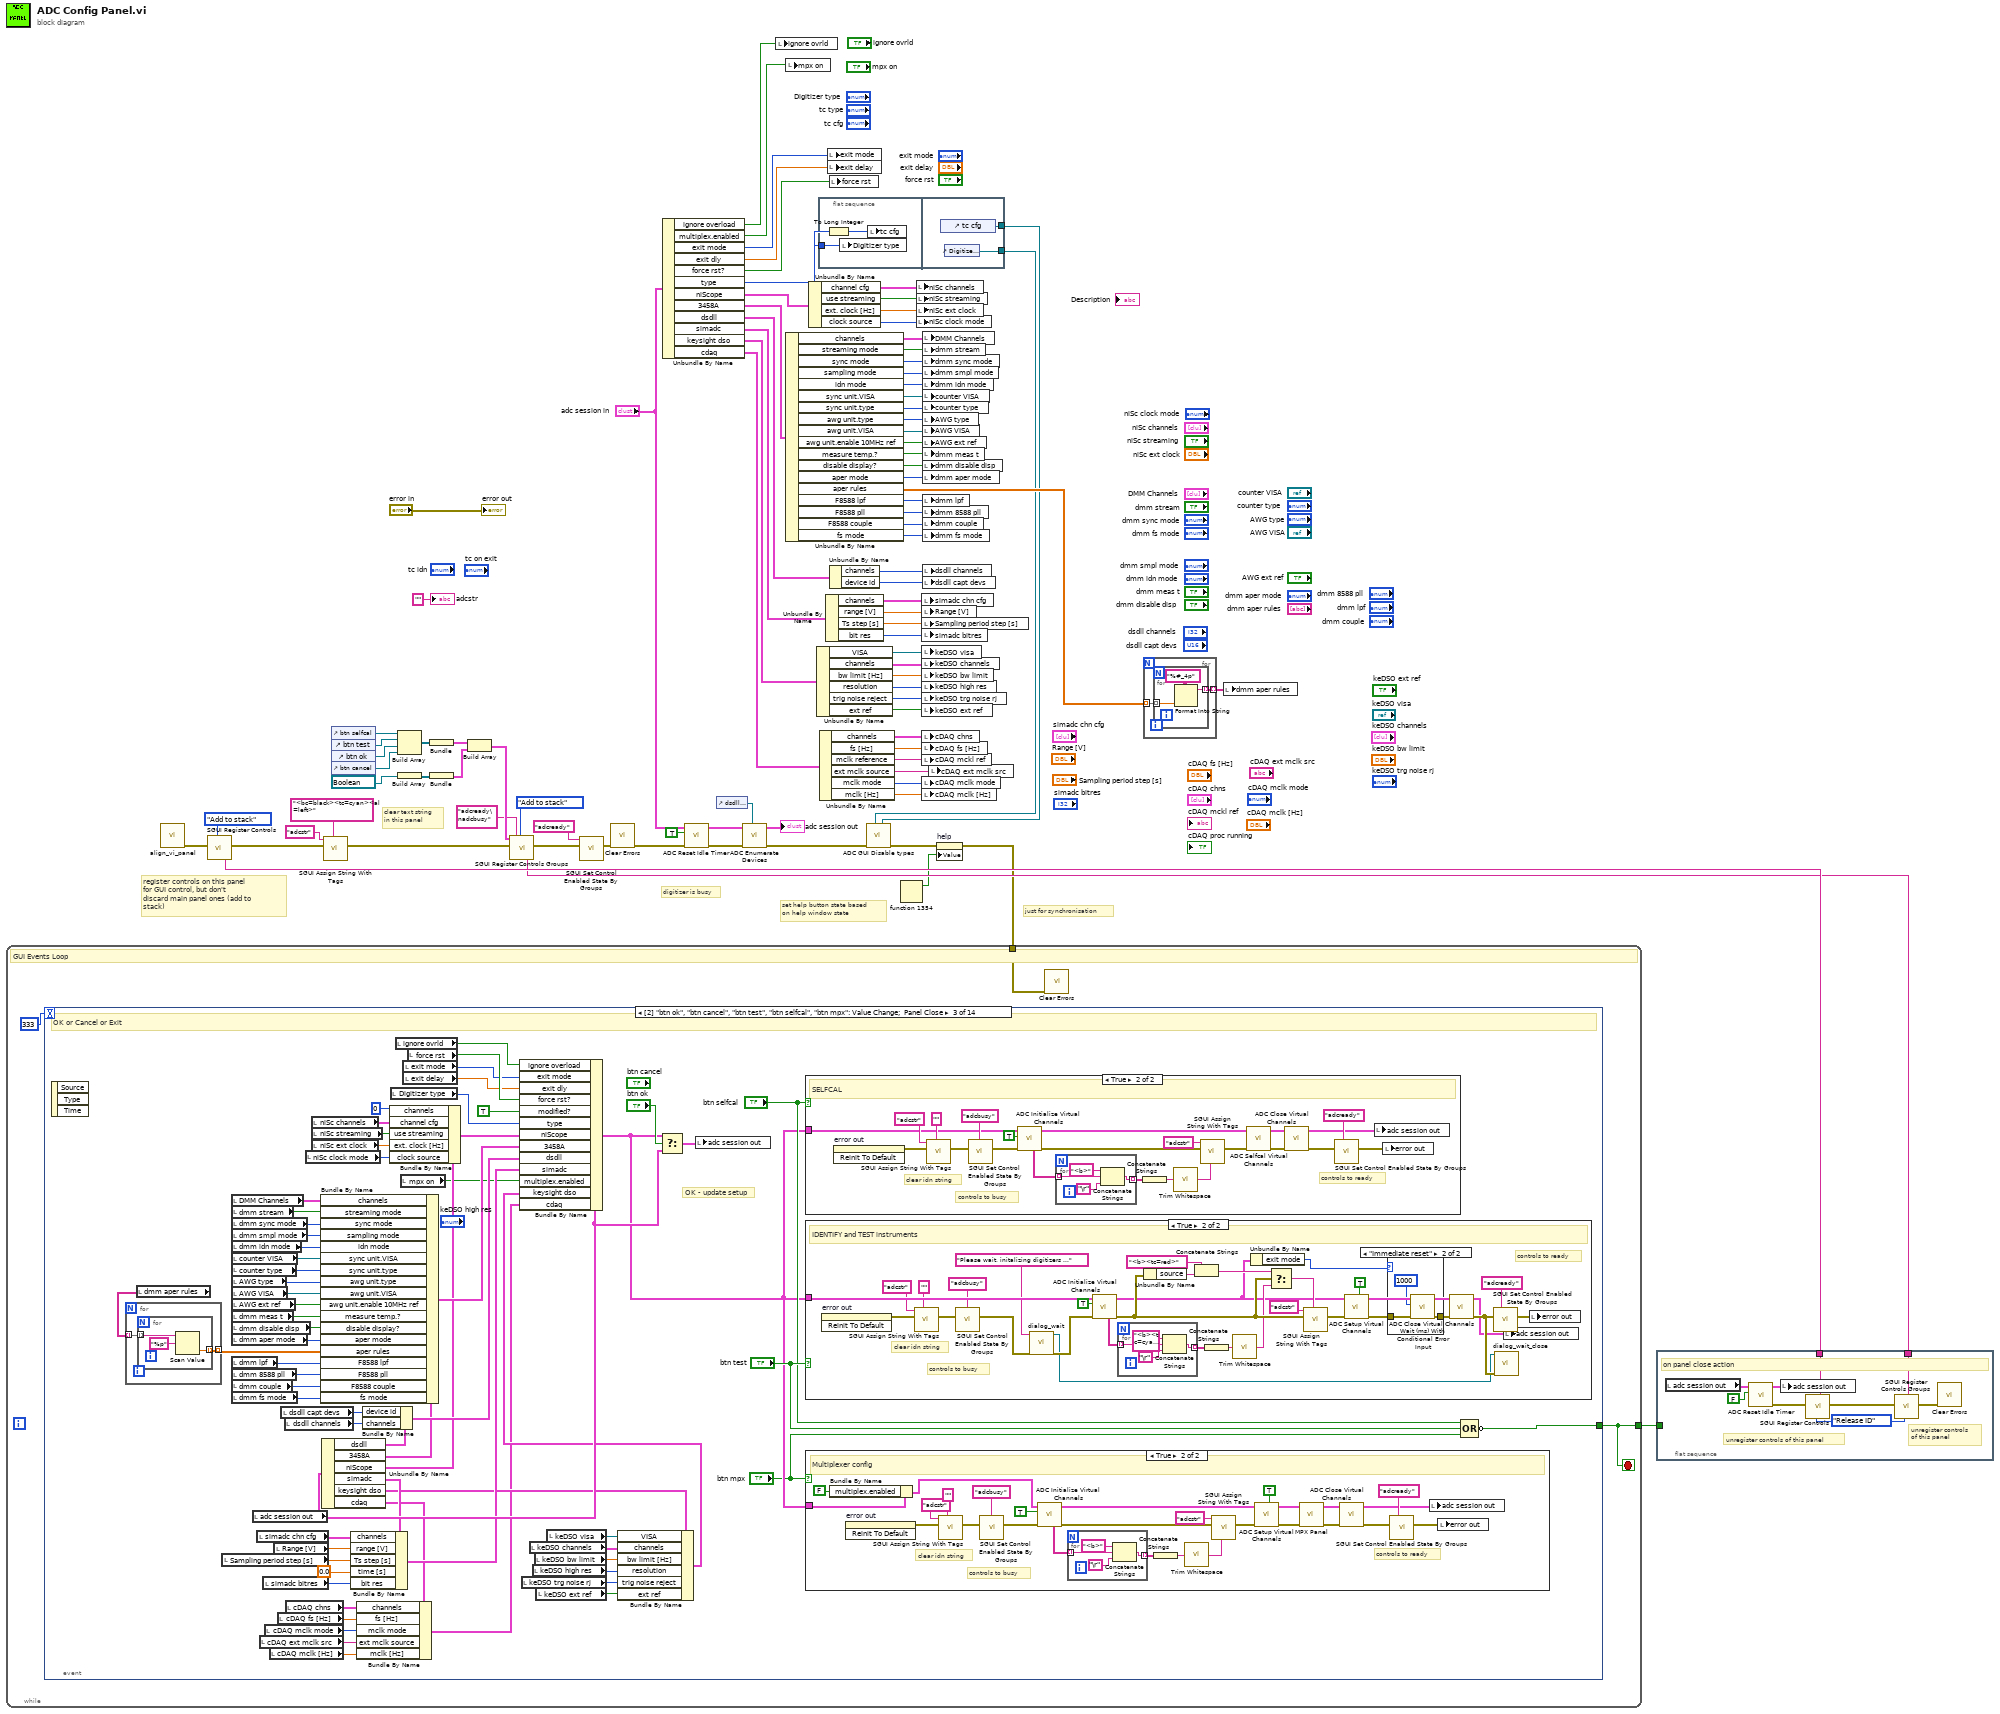
[diagram p0: block diagram]
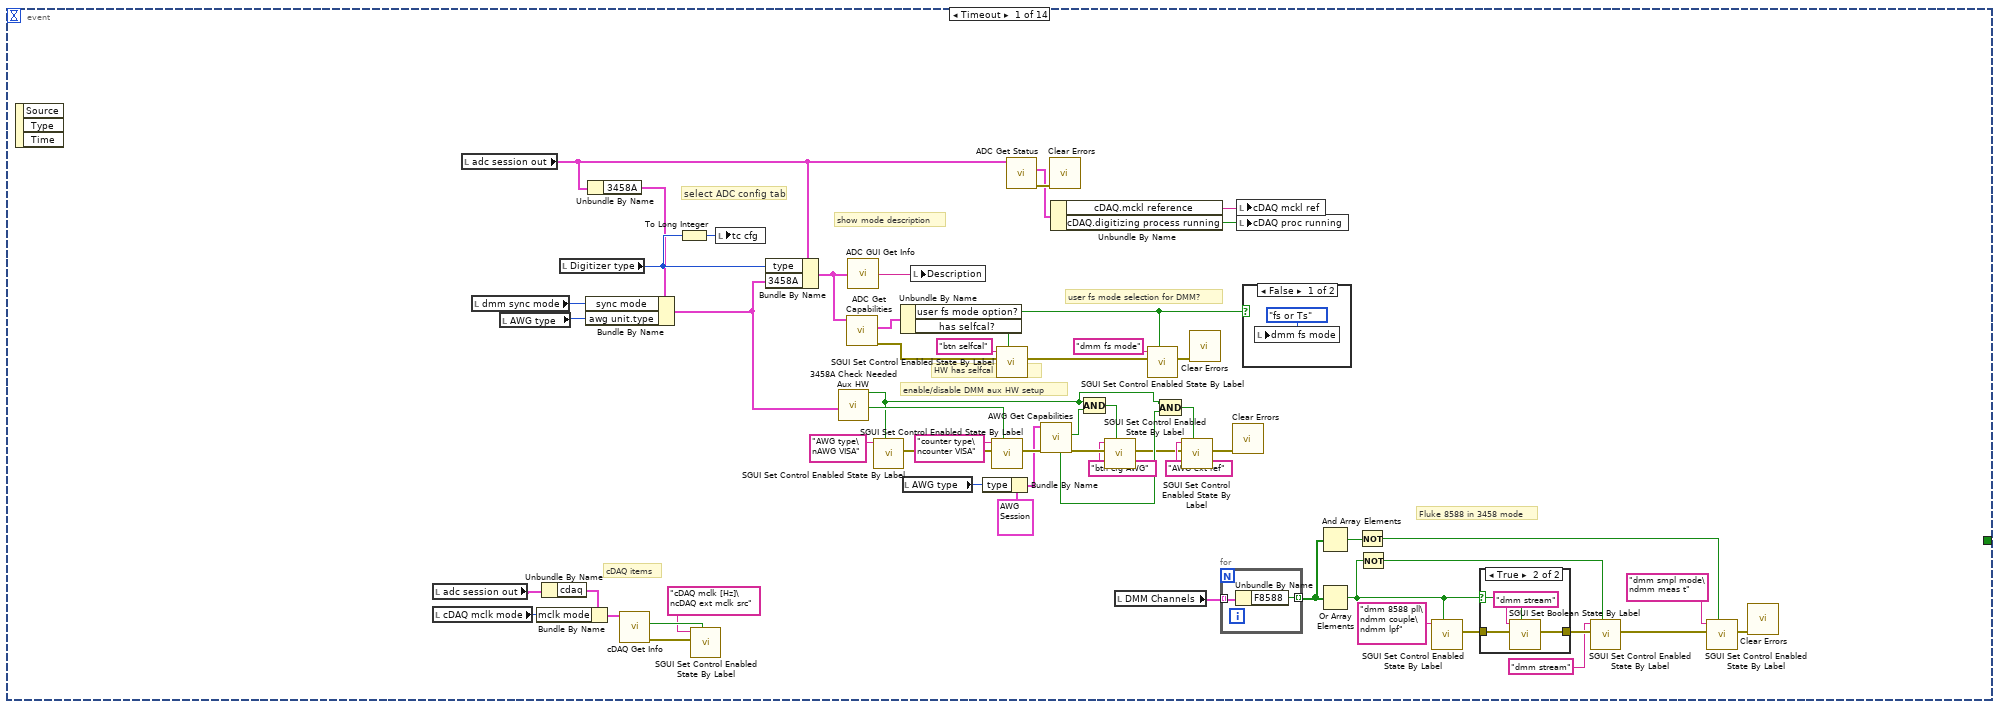
[diagram p2: hidden frame]
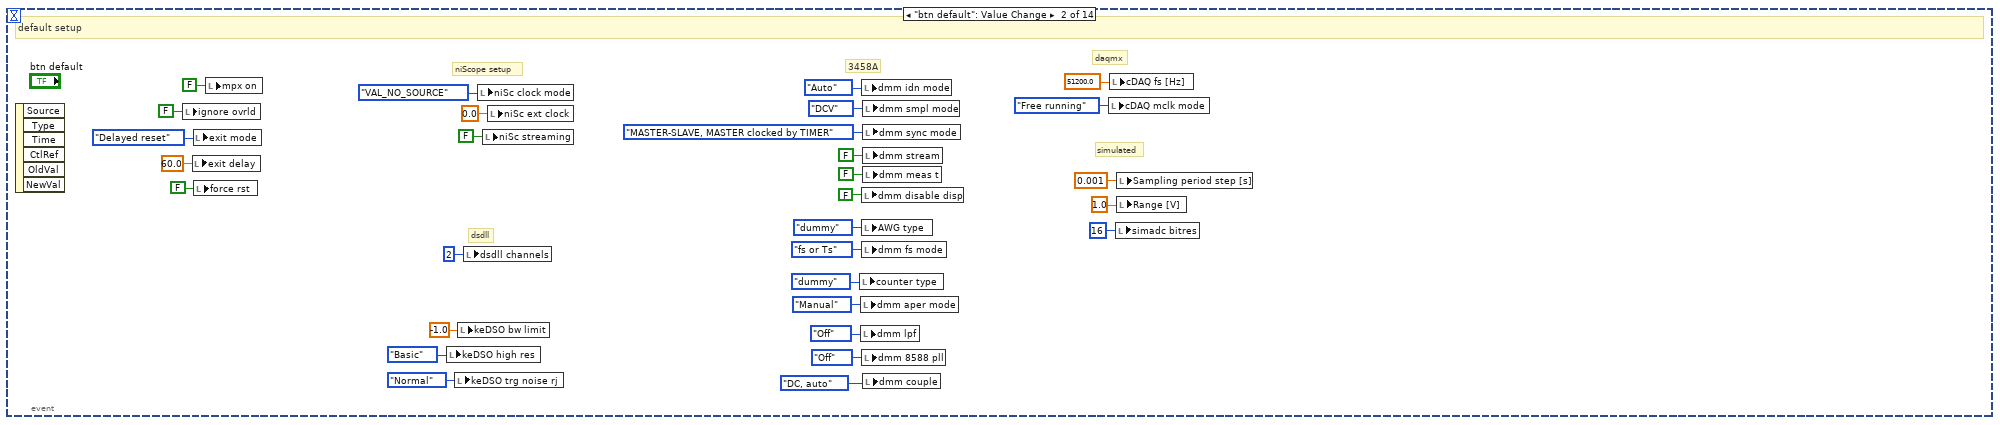
[diagram p5: hidden frame]
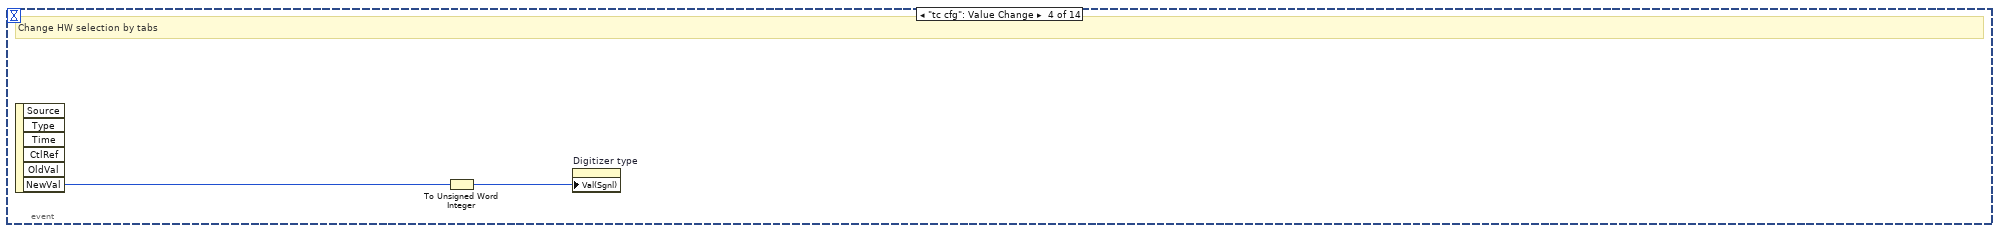
[diagram p10: hidden frame]
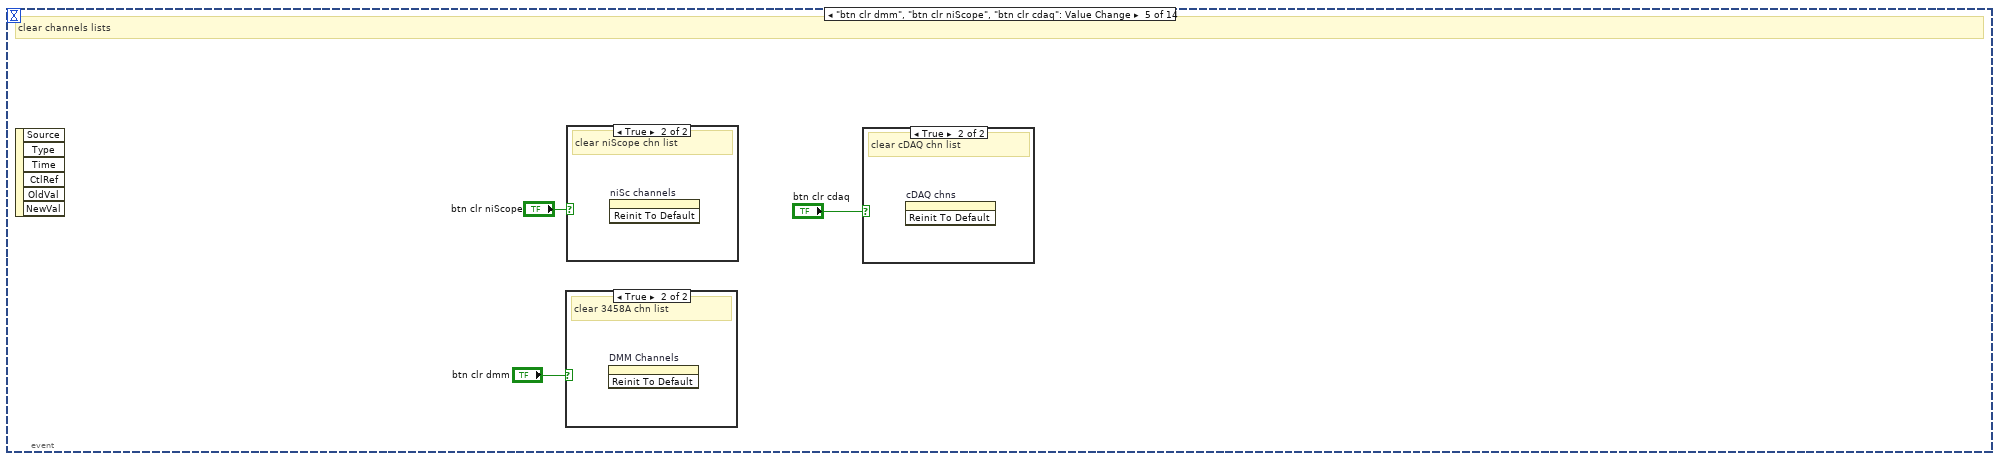
[diagram p11: hidden frame]
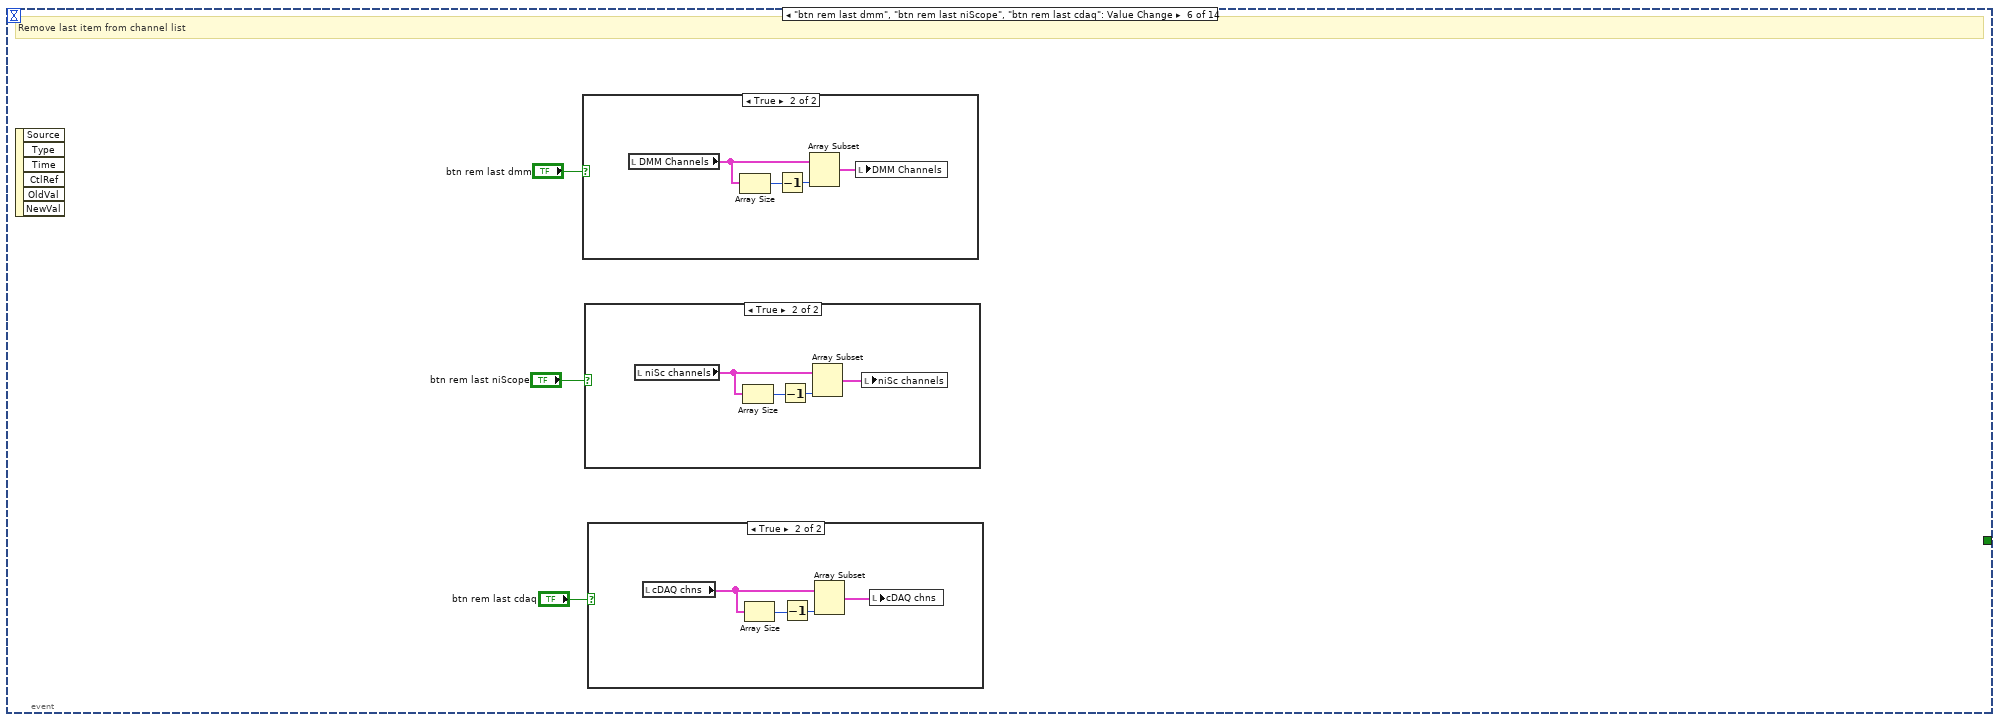
[diagram p15: hidden frame]
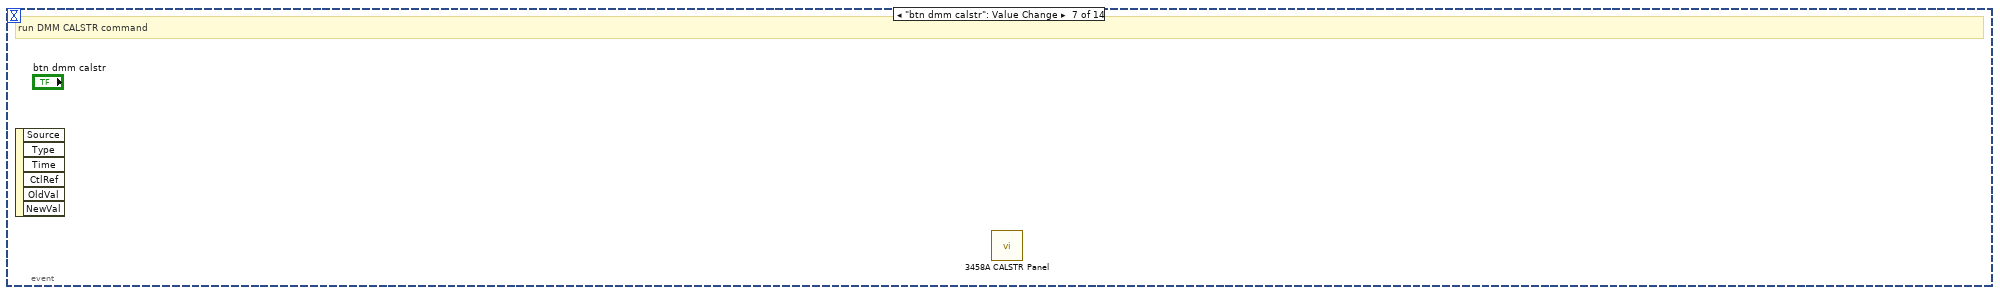
[diagram p19: hidden frame]
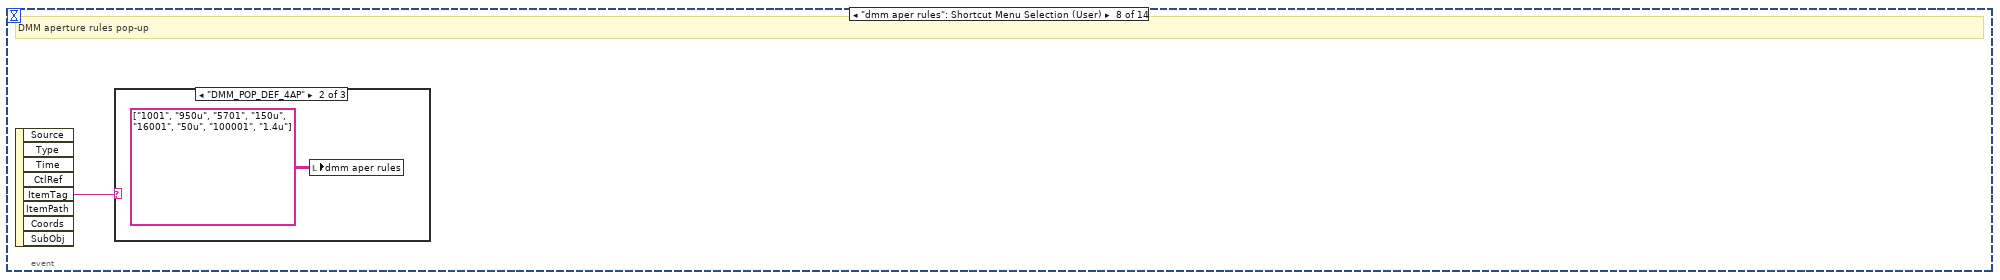
[diagram p20: hidden frame]
diagram:
  # "set help button state based\non help window state"
  # "digitizer is busy"
  # "just for synchronisation"
  # "clear text string\nin this panel"
  # "register controls on this panel\nfor GUI control, but don't\ndiscard main panel ones (add to stack)"
  n1 = call "align_vi_panel.vi"() -> ("error out"=w47:errorcluster)  [unwired: 11 in]
  n2 = call "SGUI Register Controls.vi"("error in"=w47, "register mode (overwrite)"=SGUI_Assign_References_Mode."Add to stack") -> ("assigned ID"=w40:string, "error out"=w75:errorcluster)  [unwired: 15 in, 1 out]
  n3 = call-poly "SGUI Assign String With Tags.vi"("error in"=w75, "label(s) (empty)"="adcstr" ("string (empty)"), "string (empty)"="<bc=black><tc=cyan><al=left>" ("label(s) (empty)")) -> ("error out"=w71:errorcluster)  [unwired: 7 in, 1 out]
  n4 = control-ref of="btn selfcal"() -> (w65:refnum<vi>)
  n5 = control-ref of="btn test"() -> (w64:refnum<vi>)
  n6 = control-ref of="btn ok"() -> (w63:refnum<vi>)
  n7 = control-ref of="btn cancel"() -> (w62:refnum<vi>)
  n8 = Build Array(w65, w64, w63, w62) -> (w69:refnum<vi>[])
  n9 = Build Array(refnum<vi> refnum ("btn cancel")) -> (w67:refnum<vi>[])
  n10 = Bundle(w69) -> (w70:cluster{refnum<vi>[]})  [unwired: 1 in]
  n11 = Bundle(w67) -> (w68:cluster{refnum<vi>[]})  [unwired: 1 in]
  n12 = Build Array(w70, w68) -> (w66:cluster{refnum<vi>[]}[])
  n13 = call "SGUI Register Controls Groups.vi"("control groups"=w66, "error in"=w71, "groups names"="adcready\nadcbusy", "register mode (overwrite)"=SGUI_Assign_References_Mode."Add to stack") -> ("assigned ID"=w39:string, "error out"=w58:errorcluster)  [unwired: 14 in]
  n14 = call "SGUI Set Control Enabled State By Groups.vi"("error in"=w58, "group name to enable (none)"="adcready") -> ("error out"=w56:errorcluster)  [unwired: 8 in, 1 out]
  n15 = call <vilib>:"Clear Errors.vi"("error in (no error)"=w56) -> ("error out"=w35:errorcluster)  [unwired: 5 in, 1 out]
  n16 = Unbundle By Name("adc session in") -> ("ignore overload"=w6:bool, "multiplex.enabled"=w23:bool, "exit mode"=w36:T1, "exit dly"=w37:dbl, "force rst?"=w38:bool, "type"=w55:T57, "niScope"=w92:T3, "3458A"=w88:T14, "dsdll"=w52:T53, "simadc"=w46:T58, "keysight dso"=w22:T72, "cdaq"=w16:T77)
  n17 = call "ADC Reset Idle Timer.vi"("error in"=w35, "set busy (False)"=TRUE, "adc session in"="adc session in") -> ("error out"=w34:errorcluster, "adc session out"=w32:T2)  [unwired: 7 in]
  n18 = control-ref of="dsdll capt devs"() -> (w54:refnum<vi>)
  n19 = call "ADC Enumerate Devices.vi"("capture devices ring ref"=w54, "error in"=w34, "adc session in"=w32) -> ("error out"=w27:errorcluster, "adc session out"=→"adc session out":T2)  [unwired: 7 in]
  n20 = local write "ignore ovrld"(w6) -> ()
  n21 = local write "mpx on"(w23) -> ()
  n22 = Unbundle By Name(w88) -> ("channels"=w87:T15[], "streaming mode"=w86:bool, "sync mode"=w85:T37, "sampling mode"=w84:T39, "idn mode"=w83:T38, "sync unit.VISA"=w82:refnum<visa-resource-name>, "sync unit.type"=w81:T17, "awg unit.type"=w80:T19, "awg unit.VISA"=w79:refnum<visa-resource-name>, "awg unit.enable 10MHz ref"=w78:bool, "measure temp.?"=w48:bool, "disable display?"=w41:bool, "aper mode"=w30:T45, "aper rules"=w28:dbl[][], "F8588 lpf"=w12:T47, "F8588 pll"=w11:T48, "F8588 couple"=w10:T49, "fs mode"=w5:T52)
  n23 = Unbundle By Name(w92) -> ("channel cfg"=w91:T4[], "use streaming"=w90:bool, "ext. clock [Hz]"=w89:dbl, "clock source"=w24:T13)
  n24 = Unbundle By Name(w22) -> ("VISA"=w21:refnum<visa-resource-name>, "channels"=w20:T73[], "bw limit [Hz]"=w19:dbl, "resolution"=w18:T74, "trig noise reject"=w17:enum16{"Normal", "High Sensitivity"}, "ext ref"=w1:bool)
  n25 = flat-sequence {
    tunnel: w55 -> [w93]
    tunnel: [w96] -> w26
    tunnel: [w95] -> w25
    frame #0 {
      n26 = To Long Integer(number=w93) -> (32bit integer=w94:i32)
      n27 = local write "Digitizer type"(w93) -> ()
      n28 = local write "tc cfg"(w94) -> ()
    }
    frame #1 {
      n29 = control-ref of="tc cfg"() -> (w95:refnum<vi>)
      n30 = control-ref of="Digitizer type"() -> (w96:refnum<vi>)
    }
  }
  n31 = Unbundle By Name(w16) -> ("channels"=w15:T78[], "fs [Hz]"=w14:dbl, "mclk reference"=w13:string, "ext mclk source"=w9:tag, "mclk mode"=w8:T79, "mclk [Hz]"=w7:dbl)
  n32 = Unbundle By Name(w46) -> ("channels"=w45:T59[], "range [V]"=w44:dbl, "Ts step [s]"=w43:dbl, "bit res"=w42:i32)
  n33 = local write "exit mode"(w36) -> ()
  n34 = local write "exit delay"(w37) -> ()
  n35 = local write "force rst"(w38) -> ()
  n36 = Unbundle By Name(w52) -> ("channels"=w51:i32, "device id"=w50:i32)
  n37 = call "ADC GUI Disable types.vi"("Tab ref"=w25, "Enum ref"=w26, "error in (no error)"=w27) -> ("error out"=w4:errorcluster)  [unwired: 8 in]
  n38 = fn#1354() -> (1:w3:bool)  [unwired: 1 out]
  n39 = local write "niSc channels"(w91) -> ()
  n40 = local write "niSc streaming"(w90) -> ()
  n41 = local write "niSc ext clock"(w89) -> ()
  n42 = local write "niSc clock mode"(w24) -> ()
  n43 = local write "simadc chn cfg"(w45) -> ()
  n44 = local write "Range [V]"(w44) -> ()
  n45 = local write "Sampling period step [s]"(w43) -> ()
  n46 = local write "simadc bitres"(w42) -> ()
  n47 = local write "keDSO visa"(w21) -> ()
  n48 = local write "keDSO channels"(w20) -> ()
  n49 = local write "keDSO bw limit"(w19) -> ()
  n50 = local write "keDSO high res"(w18) -> ()
  n51 = local write "keDSO trg noise rj"(w17) -> ()
  n52 = local write "keDSO ext ref"(w1) -> ()
  n53 = local write "cDAQ chns"(w15) -> ()
  n54 = local write "cDAQ fs [Hz]"(w14) -> ()
  n55 = local write "cDAQ mckl ref"(w13) -> ()
  n56 = local write "cDAQ mclk mode"(w8) -> ()
  n57 = local write "cDAQ mclk [Hz]"(w7) -> ()
  n58 = local write "DMM Channels"(w87) -> ()
  n59 = local write "dmm stream"(w86) -> ()
  n60 = local write "dmm sync mode"(w85) -> ()
  n61 = local write "dmm smpl mode"(w84) -> ()
  n62 = local write "dmm idn mode"(w83) -> ()
  n63 = local write "counter VISA"(w82) -> ()
  n64 = local write "counter type"(w81) -> ()
  n65 = local write "AWG type"(w80) -> ()
  n66 = local write "AWG VISA"(w79) -> ()
  n67 = local write "AWG ext ref"(w78) -> ()
  n68 = local write "dmm meas t"(w48) -> ()
  n69 = local write "dmm disable disp"(w41) -> ()
  n70 = local write "dmm aper mode"(w30) -> ()
  n71 = local write "dmm lpf"(w12) -> ()
  n72 = local write "dmm 8588 pll"(w11) -> ()
  n73 = local write "dmm couple"(w10) -> ()
  n74 = local write "dmm fs mode"(w5) -> ()
  n75 = local write "dsdll channels"(w51) -> ()
  n76 = local write "dsdll capt devs"(w50) -> ()
  n77 = local write "cDAQ ext mclk src"(w9) -> ()
  n78 = property on="help" class="Bool (strict)"(error in=w4, "Value"=w3) -> (error out=w2:errorcluster)  [unwired: 1 in, 1 out]
  n79 = while {
    tunnel: w2 -> [w97]
    tunnel: [w98] -> w74
    stop <- w98 stop-if-true
    # "GUI Events Loop"
    n80 = event shown="[2] \"btn ok\", \"btn cancel\", \"btn test\", \"btn selfcal\", \"btn mpx\": Value Change;  Panel Close" {
      selector: _ -> [_ _ _ _ _ _ _ _ _ _ _ _ _ _]
      dyn-events: _ -> [_ _ _ _ _ _ _ _ _ _ _ _ _ _]
      timeout: 333 -> [_ _ _ _ _ _ _ _ _ _ _ _ _ _]
      tunnel: [_ _ w247 _ _ _ _ _ _ _ _ _ _ _] -> w98
      event Timeout {
        # "user fs mode selection for DMM?"
        # "cDAQ items"
        # "Fluke 8588 in 3458 mode"
        # "enable/disable DMM aux HW setup"
        # "HW has selfcal option?"
        # "select ADC config tab"
        # "show mode description"
        n81 = event-data() -> ()  [unwired: 1 in, 3 out]
        n82 = local read "adc session out"() -> (w119:T2)
        n83 = local read "cDAQ mclk mode"() -> (w117:T79)
        n84 = local read "adc session out"() -> (w102:T2)
        n85 = local read "dmm sync mode"() -> (w158:T37)
        n86 = local read "AWG type"() -> (w100:T19)
        n87 = Unbundle By Name(w119) -> ("cdaq"=w118:T77)
        n88 = Bundle By Name(cluster=w118, "mclk mode"=w117) -> (w120:T77)
        n89 = local read "Digitizer type"() -> (w156:T57)
        n90 = Unbundle By Name(w102) -> ("3458A"=w101:T14)
        n91 = Bundle By Name(cluster=w101, "sync mode"=w158, "awg unit.type"=w100) -> (w113:T14)
        n92 = call "cDAQ Get Info.vi"("cdaq session"=w120) -> ("error out"=w116:errorcluster, "needs ext. mclk source?"=w115:bool)  [unwired: 9 in]
        n93 = To Long Integer(number=w156) -> (32bit integer=w155:i32)
        n94 = call "SGUI Set Control Enabled State By Label.vi"("error in"=w116, "labels (empty)"="cDAQ mclk [Hz]\ncDAQ ext mclk src", "Enabled? (False)"=w115) -> ()  [unwired: 7 in, 2 out]
        n95 = local write "tc cfg"(w155) -> ()
        n96 = Bundle By Name(cluster=w102, "type"=w156, "3458A"=w113) -> (w154:T2)
        n97 = call "3458A Check Needed Aux HW.vi"("digitizer session"=w113) -> ("uses AWG clocking?"=w110:bool, "uses counter?"=w147:bool)  [unwired: 13 in, 4 out]
        n98 = call "ADC Get Capabilities.vi"("adc session in"=w154) -> ("error out"=w150:errorcluster, "capabilities"=w153:T82)  [unwired: 8 in, 1 out]
        n99 = call "ADC GUI Get Info.vi"("adc session"=w154) -> ("configuration description"=w157:string)
        n100 = call "SGUI Set Control Enabled State By Label.vi"("labels (empty)"="AWG type\nAWG VISA", "Enabled? (False)"=w110) -> ("error out"=w148:errorcluster)  [unwired: 8 in, 1 out]
        n101 = Unbundle By Name(w153) -> ("user fs mode option?"=w103:bool, "has selfcal?"=w152:bool)
        n102 = local read "AWG type"() -> (w121:T19)
        n103 = local write "Description"(w157) -> ()
        n104 = Bundle By Name(cluster=T18 {"type"=enum."Agilent 331xxA to 332xxA", "VISA"="", "enable 10MHz ref"=FALSE, "cmi ckd2"={"VISA"="", "clock source"=enum."Auto", "manual ref clk"=FALSE, "ref clock [Hz]"=0.0, "div mode"=enum."Set divisor directly"}, "cmi sync v3"={"VISA"="", "baud rate [bd/s]"=115200, "source"=enum."Auto", "hv range"=enum."1kV", "fsrc is fixed"=FALSE, "fsrc [Hz]"=10000000.0, "freq integ [s]"=1.0, "freq filter"=5, "trig level"=enum."TTL 5V", "chn1 mode"=enum."Source divider", "chn1 level"=enum."Positive 5V", "chn2 mode"=enum."Source divider", "chn2 level"=enum."Positive 5V", "chn2 div"=1, "chn3 mode"=enum."Chn 1 Active", "chn3 level"=enum."Positive 5V", "chn1 div entry"=enum."Calculate nearest divisor from measured fx", "chn1 dev limit [%]"=1.0, "chn1 check dev"=FALSE}, "trigger"={"source"=enum."Immediate", "slope"=enum."POS", "coupling"=enum."DC", "level [V]"=0.0, "hysteresis [V]"=0.0, "pre-trigger [%]"=0.0}, "HMF2500 cfg"={"Baud Rate"=9600, "Parity"=0, "Data Bits"=8, "Flow Control"=4}} ("awg session"), "type"=w121) -> (w123:T18)
        n105 = call "SGUI Set Control Enabled State By Label.vi"("error in"=w148, "labels (empty)"="counter type\ncounter VISA", "Enabled? (False)"=w147) -> ("error out"=w126:errorcluster)  [unwired: 7 in, 1 out]
        n106 = call "SGUI Set Control Enabled State By Label.vi"("error in"=w150, "labels (empty)"="btn selfcal", "Enabled? (False)"=w152) -> ("error out"=w105:errorcluster)  [unwired: 7 in, 1 out]
        n107 = call "ADC Get Status.vi"("adc session in"=w102) -> ("error out"=w145:errorcluster, "status"=w144:T84)  [unwired: 8 in, 1 out]
        n108 = call "AWG Get Capabilities.vi"("error in (no error)"=w126, "awg session"=w123) -> ("error out"=w128:errorcluster, "has cfg panel?"=w125:bool, "has ext ref?"=w109:bool)  [unwired: 5 in, 2 out]
        n109 = call <vilib>:"Clear Errors.vi"("error in (no error)"=w145) -> ()  [unwired: 5 in, 2 out]
        n110 = Unbundle By Name(w144) -> ("cDAQ.mckl reference"=w143:string, "cDAQ.digitizing process running"=w142:bool)
        n111 = Compound Arithmetic op=AND(w110, w125) -> (w124:bool)
        n112 = call "SGUI Set Control Enabled State By Label.vi"("error in"=w128, "labels (empty)"="btn cfg AWG", "Enabled? (False)"=w124) -> ("error out"=w107:errorcluster)  [unwired: 7 in, 1 out]
        n113 = local read "DMM Channels"() -> (w141:T15[])
        n114 = call "SGUI Set Control Enabled State By Label.vi"("error in"=w105, "labels (empty)"="dmm fs mode", "Enabled? (False)"=w103) -> ("error out"=w104:errorcluster)  [unwired: 7 in, 1 out]
        n115 = Compound Arithmetic op=AND(w110, w109) -> (w108:bool)
        n116 = call "SGUI Set Control Enabled State By Label.vi"("error in"=w107, "labels (empty)"="AWG ext ref", "Enabled? (False)"=w108) -> ("error out"=w111:errorcluster)  [unwired: 7 in, 1 out]
        n117 = call <vilib>:"Clear Errors.vi"("error in (no error)"=w104) -> ()  [unwired: 5 in, 2 out]
        n118 = for {
          tunnel: w141 -> [w166] mode=indexing
          tunnel: [w165] -> w140 mode=indexing
          n119 = Unbundle By Name(w166) -> ("F8588"=w165:bool)
        }
        n120 = call <vilib>:"Clear Errors.vi"("error in (no error)"=w111) -> ()  [unwired: 5 in, 2 out]
        n121 = local write "cDAQ mckl ref"(w143) -> ()
        n122 = local write "cDAQ proc running"(w142) -> ()
        n123 = case shown="False" w103 {
          frame False {
            n124 = local write "dmm fs mode"(3458A_Sample_Rate_Mode."fs or Ts" ("dmm fs mode")) -> ()
          }
          frame True {
          }
        }
        n125 = And Array Elements(Boolean array=w140) -> (logical AND=w138:bool)
        n126 = Or Array Elements(Boolean array=w140) -> (logical OR=w131:bool)
        n127 = Not(x=w138) -> (.not. x?=w137:bool)
        n128 = Not(x=w131) -> (.not. x?=w130:bool)
        n129 = call "SGUI Set Control Enabled State By Label.vi"("labels (empty)"="dmm 8588 pll\ndmm couple\ndmm lpf", "Enabled? (False)"=w131) -> ("error out"=w134:errorcluster)  [unwired: 8 in, 1 out]
        n130 = case shown="True" w131 {
          selector: w131 -> [_ w163]
          tunnel: w134 -> [w160 w164]
          tunnel: [w160 w161] -> w133
          frame False {
          }
          frame True {
            n131 = call "SGUI Set Boolean State By Label.vi"("binary state in (False)"=w163, "error in"=w164, "control label(s) ('btn stop')"="dmm stream" ("labels (empty)")) -> ("error out"=w161:errorcluster)  [unwired: 7 in, 1 out]
          }
        }
        n132 = call "SGUI Set Control Enabled State By Label.vi"("error in"=w133, "labels (empty)"="dmm stream", "Enabled? (False)"=w130) -> ("error out"=w129:errorcluster)  [unwired: 7 in, 1 out]
        n133 = call "SGUI Set Control Enabled State By Label.vi"("error in"=w129, "labels (empty)"="dmm smpl mode\ndmm meas t", "Enabled? (False)"=w137) -> ("error out"=w136:errorcluster)  [unwired: 7 in, 1 out]
        n134 = call <vilib>:"Clear Errors.vi"("error in (no error)"=w136) -> ()  [unwired: 5 in, 2 out]
      }
      event "btn default": Value Change {
        # "daqmx"
        # "simulated"
        # "dsdll"
        # "3458A"
        # "niScope setup"
        # "default setup"
        n135 = event-data() -> ()  [unwired: 1 in, 6 out]
        n136 = local write "ignore ovrld"(FALSE ("ignore ovrld")) -> ()
        n137 = local write "exit delay"(60.0 ("exit delay")) -> ()
        n138 = local write "exit mode"(ADC_On_Close_Action."Delayed reset" ("exit mode")) -> ()
        n139 = local write "force rst"(FALSE ("force rst")) -> ()
        n140 = local write "mpx on"(FALSE ("mpx on")) -> ()
        n141 = local write "keDSO high res"(KeDSO_High_Resolution_Mode."Basic" ("keDSO high res")) -> ()
        n142 = local write "keDSO trg noise rj"(enum16{"Normal", "High Sensitivity"}."Normal" ("keDSO trg noise rj")) -> ()
        n143 = local write "keDSO bw limit"(-1.0 ("keDSO bw limit")) -> ()
        n144 = local write "dsdll channels"(2 ("dsdll channels")) -> ()
        n145 = local write "niSc clock mode"(niScope_Reference_Clock."VAL_NO_SOURCE" ("niSc clock mode")) -> ()
        n146 = local write "niSc streaming"(FALSE ("niSc streaming")) -> ()
        n147 = local write "niSc ext clock"(0.0 ("niSc ext clock")) -> ()
        n148 = local write "counter type"(Counter_Type."dummy" ("counter type")) -> ()
        n149 = local write "dmm aper mode"(3458A_Aperture_Selection_Mode."Manual" ("dmm aper mode")) -> ()
        n150 = local write "dmm lpf"(F8588A_Low_Pass_Filter."Off" ("dmm lpf")) -> ()
        n151 = local write "dmm idn mode"(3458A_Idn_Mode."Auto" ("dmm idn mode")) -> ()
        n152 = local write "dmm disable disp"(FALSE ("dmm disable disp")) -> ()
        n153 = local write "AWG type"(AWG_Type."dummy" ("AWG type")) -> ()
        n154 = local write "dmm fs mode"(3458A_Sample_Rate_Mode."fs or Ts" ("dmm fs mode")) -> ()
        n155 = local write "dmm 8588 pll"(F8588A_Phase_Lock."Off" ("dmm 8588 pll")) -> ()
        n156 = local write "dmm smpl mode"(Sampling_Mode."DCV" ("dmm smpl mode")) -> ()
        n157 = local write "dmm sync mode"(3458A_Sync_Mode."MASTER-SLAVE, MASTER clocked by TIMER" ("dmm sync mode")) -> ()
        n158 = local write "dmm stream"(FALSE ("dmm stream")) -> ()
        n159 = local write "dmm meas t"(FALSE ("dmm meas t")) -> ()
        n160 = local write "dmm couple"(F8588A_Coupling."DC, auto" ("dmm couple")) -> ()
        n161 = local write "cDAQ mclk mode"(cDAQ_Master_Clock_Mode."Free running" ("cDAQ mclk mode")) -> ()
        n162 = local write "cDAQ fs [Hz]"(51200.0 ("cDAQ fs [Hz]")) -> ()
        n163 = local write "simadc bitres"(16 ("simadc bitres")) -> ()
        n164 = local write "Sampling period step [s]"(0.001 ("Sampling period step [s]")) -> ()
        n165 = local write "Range [V]"(1.0 ("Range [V]")) -> ()
      }
      event "btn ok", "btn cancel", "btn test", "btn selfcal", "btn mpx": Value Change; Panel Close {
        # "OK - update setup"
        # "OK or Cancel or Exit"
        n166 = event-data() -> ()  [unwired: 1 in, 3 out]
        n167 = local read "dmm aper rules"() -> (w222:string[][])
        n168 = for {
          tunnel: w222 -> [w298] mode=indexing
          tunnel: [w297] -> w221 mode=indexing
          n169 = for {
            tunnel: w298 -> [w301] mode=indexing
            tunnel: [w300] -> w297 mode=indexing
            n170 = Scan Value(string=w301, format string="%p") -> (value=w300:dbl)  [unwired: 1 in, 1 out]
          }
        }
        n171 = local read "Sampling period step [s]"() -> (w231:dbl)
        n172 = local read "DMM Channels"() -> (w262:T15[])
        n173 = local read "dmm stream"() -> (w261:bool)
        n174 = local read "dmm sync mode"() -> (w260:T37)
        n175 = local read "dmm smpl mode"() -> (w259:T39)
        n176 = local read "dmm idn mode"() -> (w258:T38)
        n177 = local read "counter VISA"() -> (w257:refnum<visa-resource-name>)
        n178 = local read "counter type"() -> (w256:T17)
        n179 = local read "AWG type"() -> (w255:T19)
        n180 = local read "AWG VISA"() -> (w254:refnum<visa-resource-name>)
        n181 = local read "AWG ext ref"() -> (w253:bool)
        n182 = local read "dmm meas t"() -> (w237:bool)
        n183 = local read "dmm disable disp"() -> (w227:bool)
        n184 = local read "dmm aper mode"() -> (w223:T45)
        n185 = local read "dmm lpf"() -> (w205:T47)
        n186 = local read "dmm 8588 pll"() -> (w204:T48)
        n187 = local read "dmm couple"() -> (w203:T49)
        n188 = local read "dmm fs mode"() -> (w198:T52)
        n189 = local read "adc session out"() -> (w242:T2)
        n190 = local read "simadc chn cfg"() -> (w233:T59[])
        n191 = local read "cDAQ ext mclk src"() -> (w201:tag)
        n192 = local read "simadc bitres"() -> (w228:i32)
        n193 = local read "cDAQ mclk mode"() -> (w202:T79)
        n194 = local read "cDAQ mclk [Hz]"() -> (w200:dbl)
        n195 = local read "Range [V]"() -> (w232:dbl)
        n196 = local read "cDAQ fs [Hz]"() -> (w207:dbl)
        n197 = local read "dsdll capt devs"() -> (w244:u16)
        n198 = local read "dsdll channels"() -> (w243:i32)
        n199 = local read "cDAQ chns"() -> (w208:T78[])
        n200 = local read "niSc clock mode"() -> (w220:T13)
        n201 = local read "niSc channels"() -> (w265:T4[])
        n202 = local read "niSc streaming"() -> (w264:bool)
        n203 = local read "niSc ext clock"() -> (w263:dbl)
        n204 = Unbundle By Name(w242) -> ("dsdll"=w241:T53, "3458A"=w240:T14, "niScope"=w239:T3, "simadc"=w234:T58, "keysight dso"=w216:T72, "cdaq"=w209:T77)
        n205 = Bundle By Name(cluster=w240, "channels"=w262, "streaming mode"=w261, "sync mode"=w260, "sampling mode"=w259, "idn mode"=w258, "sync unit.VISA"=w257, "sync unit.type"=w256, "awg unit.type"=w255, "awg unit.VISA"=w254, "awg unit.enable 10MHz ref"=w253, "measure temp.?"=w237, "disable display?"=w227, "aper mode"=w223, "aper rules"=w221, "F8588 lpf"=w205, "F8588 pll"=w204, "F8588 couple"=w203, "fs mode"=w198) -> (w251:T14)
        n206 = Bundle By Name(cluster=w234, "channels"=w233, "range [V]"=w232, "Ts step [s]"=w231, "time [s]"=0.0, "bit res"=w228) -> (w229:T58)
        n207 = Bundle By Name(cluster=w209, "channels"=w208, "fs [Hz]"=w207, "mclk mode"=w202, "ext mclk source"=w201, "mclk [Hz]"=w200) -> (w206:T77)
        n208 = Bundle By Name(cluster=w241, "device id"=w244, "channels"=w243) -> (w245:T53)
        n209 = Bundle By Name(cluster=w239, "channels"=0, "channel cfg"=w265, "use streaming"=w264, "ext. clock [Hz]"=w263, "clock source"=w220) -> (w252:T3)
        n210 = local read "Digitizer type"() -> (w250:T57)
        n211 = local read "ignore ovrld"() -> (w199:bool)
        n212 = local read "mpx on"() -> (w219:bool)
        n213 = local read "exit mode"() -> (w224:T1)
        n214 = local read "exit delay"() -> (w225:dbl)
        n215 = local read "force rst"() -> (w226:bool)
        n216 = local read "keDSO trg noise rj"() -> (w211:enum16{"Normal", "High Sensitivity"})
        n217 = local read "keDSO channels"() -> (w214:T73[])
        n218 = local read "keDSO high res"() -> (w212:T74)
        n219 = local read "keDSO bw limit"() -> (w213:dbl)
        n220 = local read "keDSO ext ref"() -> (w197:bool)
        n221 = local read "keDSO visa"() -> (w215:refnum<visa-resource-name>)
        n222 = Bundle By Name(cluster=w216, "VISA"=w215, "channels"=w214, "bw limit [Hz]"=w213, "resolution"=w212, "trig noise reject"=w211, "ext ref"=w197) -> (w210:T72)
        n223 = Bundle By Name(cluster=w242, "ignore overload"=w199, "exit mode"=w224, "exit dly"=w225, "force rst?"=w226, "modified?"=TRUE, "type"=w250, "niScope"=w252, "3458A"=w251, "dsdll"=w245, "simadc"=w229, "multiplex.enabled"=w219, "keysight dso"=w210, "cdaq"=w206) -> (w218:T2)
        n224 = Select(t=w218, s="btn ok", f=w242) -> (s? t:f=w248:T2)
        n225 = local write "adc session out"(w248) -> ()
        n226 = case shown="True" "btn selfcal" {
          tunnel: w218 -> [_ w308]
          frame False {
          }
          frame True {
            # "controls to ready"
            # "controls to busy"
            # "clear idn string"
            # "SELFCAL"
            n227 = invoke on="error out" class="Clust (strict)" method="Reinit To Default"() -> (error out=w309:errorcluster)  [unwired: 3 in, 2 out]
            n228 = call-poly "SGUI Assign String With Tags.vi"("error in"=w309, "label(s) (empty)"="adcstr", "string (empty)"="") -> ("error out"=w312:errorcluster)  [unwired: 7 in, 1 out]
            n229 = call "SGUI Set Control Enabled State By Groups.vi"("error in"=w312, "group name to enable (none)"="adcbusy") -> ("error out"=w313:errorcluster)  [unwired: 8 in, 1 out]
            n230 = call "ADC Initialize Virtual Channels.vi"("error in"=w313, "Reset? (False)"=TRUE, "adc session in"=w308) -> ("error out"=w318:errorcluster, "adc session out"=w306:T2, "all instruments idn strings"=w302:string[])  [unwired: 3 in, 3 out]
            n231 = for {
              tunnel: w302 -> [w327] mode=indexing
              tunnel: [w325] -> w320 mode=indexing
              n232 = Concatenate Strings("<b>" ("string"), w327, "\r") -> (w325:string)
            }
            n233 = Concatenate Strings(w320) -> (w321:string)
            n234 = call <vilib>:"Trim Whitespace.vi"("string"=w321) -> ("trimmed string"=w322:string)  [unwired: 1 in]
            n235 = call-poly "SGUI Assign String With Tags.vi"("error in"=w318, "label(s) (empty)"="adcstr", "string (empty)"=w322) -> ("error out"=w307:errorcluster)  [unwired: 7 in, 1 out]
            n236 = call "ADC Selfcal Virtual Channels.vi"("error in"=w307, "adc session in"=w306) -> ("error out"=w304:errorcluster, "adc session out"=w305:T2)  [unwired: 8 in]
            n237 = call "ADC Close Virtual Channels.vi"("error in"=w304, "adc session in"=w305) -> ("error out"=w315:errorcluster, "adc session out"=w303:T2)  [unwired: 8 in]
            n238 = call "SGUI Set Control Enabled State By Groups.vi"("error in"=w315, "group name to enable (none)"="adcready") -> ("error out"=w316:errorcluster)  [unwired: 8 in, 1 out]
            n239 = local write "adc session out"(w303) -> ()
            n240 = local write "error out"(w316) -> ()
          }
        }
        n241 = case shown="True" "btn test" {
          tunnel: w218 -> [_ w359]
          frame False {
          }
          frame True {
            # "controls to ready"
            # "controls to busy"
            # "clear idn string"
            # "IDENTIFY and TEST instruments"
            n242 = invoke on="error out" class="Clust (strict)" method="Reinit To Default"() -> (error out=w358:errorcluster)  [unwired: 3 in, 2 out]
            n243 = call-poly "SGUI Assign String With Tags.vi"("error in"=w358, "label(s) (empty)"="adcstr", "string (empty)"="") -> ("error out"=w355:errorcluster)  [unwired: 7 in, 1 out]
            n244 = call "SGUI Set Control Enabled State By Groups.vi"("error in"=w355, "group name to enable (none)"="adcbusy") -> ("error out"=w340:errorcluster)  [unwired: 8 in, 1 out]
            n245 = call "dialog_wait.vi"("error in"=w340, "message string"="Please wait, initalizing digitizers ...") -> ("error out"=w339:errorcluster, "reference out"=w336:refnum<vi>)  [unwired: 8 in]
            n246 = call "ADC Initialize Virtual Channels.vi"("error in"=w339, "Reset? (False)"=TRUE, "adc session in"=w359) -> ("error out"=w344:errorcluster, "adc session out"=w330:T2, "all instruments idn strings"=w333:string[])  [unwired: 3 in, 3 out]
            n247 = for {
              tunnel: w333 -> [w367] mode=indexing
              tunnel: [w365] -> w350 mode=indexing
              n248 = Concatenate Strings("<b><tc=cyan>" ("string"), w367, "\r") -> (w365:string)
            }
            n249 = Unbundle By Name(w344) -> ("source"=w346:string)
            n250 = Concatenate Strings("<b><tc=red>" ("string"), w346) -> (w343:string)
            n251 = Concatenate Strings(w350) -> (w349:string)
            n252 = call <vilib>:"Trim Whitespace.vi"("string"=w349) -> ("trimmed string"=w342:string)  [unwired: 1 in]
            n253 = Unbundle By Name(w330) -> ("exit mode"=w334:T1)
            n254 = Select(t=w343, s=w344, f=w342) -> (s? t:f=w341:string)
            n255 = call-poly "SGUI Assign String With Tags.vi"("error in"=w344, "label(s) (empty)"="adcstr", "string (empty)"=w341) -> ("error out"=w332:errorcluster)  [unwired: 7 in, 1 out]
            n256 = call "ADC Setup Virtual Channels.vi"("Force valid defaults (False)"=TRUE, "error in"=w332, "adc session in"=w330) -> ("error out"=w331:errorcluster, "adc session out"=w329:T2)  [unwired: 7 in]
            n257 = case shown="\"Immediate reset\"" w334 {
              tunnel: w331 -> [w360 w362]
              tunnel: [w360 w361] -> w347
              frame Default {
              }
              frame "Immediate reset" {
                n258 = call "Wait (ms) With Conditional Error Input.vi"("error in (no error)"=w362, "milliseconds to wait"=u32 1000) -> ("error out"=w361:errorcluster)  [unwired: 8 in, 1 out]
              }
            }
            n259 = call "ADC Close Virtual Channels.vi"("error in"=w347, "adc session in"=w329) -> ("error out"=w337:errorcluster, "adc session out"=w335:T2)  [unwired: 8 in]
            n260 = call "SGUI Set Control Enabled State By Groups.vi"("error in"=w337, "group name to enable (none)"="adcready") -> ("error out"=w353:errorcluster)  [unwired: 8 in, 1 out]
            n261 = call "dialog_wait_close.vi"("error in"=w337, "async vi ref"=w336) -> ()  [unwired: 2 in]
            n262 = local write "adc session out"(w335) -> ()
            n263 = local write "error out"(w353) -> ()
          }
        }
        n264 = case shown="True" "btn mpx" {
          tunnel: w218 -> [_ w268]
          frame False {
          }
          frame True {
            # "controls to ready"
            # "controls to busy"
            # "clear idn string"
            # "Multiplexer config"
            n265 = Bundle By Name(cluster=w268, "multiplex.enabled"=FALSE) -> (w267:T2)
            n266 = invoke on="error out" class="Clust (strict)" method="Reinit To Default"() -> (error out=w278:errorcluster)  [unwired: 3 in, 2 out]
            n267 = call-poly "SGUI Assign String With Tags.vi"("error in"=w278, "label(s) (empty)"="adcstr", "string (empty)"="") -> ("error out"=w281:errorcluster)  [unwired: 7 in, 1 out]
            n268 = call "SGUI Set Control Enabled State By Groups.vi"("error in"=w281, "group name to enable (none)"="adcbusy") -> ("error out"=w282:errorcluster)  [unwired: 8 in, 1 out]
            n269 = call "ADC Initialize Virtual Channels.vi"("error in"=w282, "Reset? (False)"=TRUE, "adc session in"=w267) -> ("error out"=w287:errorcluster, "adc session out"=w271:T2, "all instruments idn strings"=w276:string[])  [unwired: 3 in, 3 out]
            n270 = for {
              tunnel: w276 -> [w296] mode=indexing
              tunnel: [w294] -> w289 mode=indexing
              n271 = Concatenate Strings("<b>" ("string"), w296, "\r") -> (w294:string)
            }
            n272 = Concatenate Strings(w289) -> (w290:string)
            n273 = call <vilib>:"Trim Whitespace.vi"("string"=w290) -> ("trimmed string"=w291:string)  [unwired: 1 in]
            n274 = call-poly "SGUI Assign String With Tags.vi"("error in"=w287, "label(s) (empty)"="adcstr", "string (empty)"=w291) -> ("error out"=w273:errorcluster)  [unwired: 7 in, 1 out]
            n275 = call "ADC Setup Virtual Channels.vi"("Force valid defaults (False)"=TRUE, "error in"=w273, "adc session in"=w271) -> ("error out"=w272:errorcluster, "adc session out"=w270:T2)  [unwired: 7 in]
            n276 = call "MPX Panel.vi"("error in"=w272, "session in"=w270) -> ("error out"=w275:errorcluster, "session out"=w274:T2)  [unwired: 8 in]
            n277 = call "ADC Close Virtual Channels.vi"("error in"=w275, "adc session in"=w274) -> ("error out"=w284:errorcluster, "adc session out"=w277:T2)  [unwired: 8 in]
            n278 = call "SGUI Set Control Enabled State By Groups.vi"("error in"=w284, "group name to enable (none)"="adcready") -> ("error out"=w285:errorcluster)  [unwired: 8 in, 1 out]
            n279 = local write "adc session out"(w277) -> ()
            n280 = local write "error out"(w285) -> ()
          }
        }
        n281 = Compound Arithmetic op=OR("btn selfcal", "btn test", "btn mpx") -> (invert w247:bool)
      }
      event "tc cfg": Value Change {
        # "Change HW selection by tabs"
        n282 = event-data() -> ("NewVal"=w369:T80)  [unwired: 1 in, 5 out]
        n283 = To Unsigned Word Integer(number=w369) -> (unsigned 16bit integer=w368:u16)
        n284 = property on="Digitizer type" class="Enum (strict)"("Val(Sgnl)"=w368) -> ()  [unwired: 2 in, 2 out]
      }
      event "btn clr dmm", "btn clr niScope", "btn clr cdaq": Value Change {
        # "clear channels lists"
        n285 = event-data() -> ()  [unwired: 1 in, 6 out]
        n286 = case shown="True" "btn clr dmm" {
          frame False {
          }
          frame True {
            # "clear 3458A chn list"
            n287 = invoke on="DMM Channels" class="Arr" method="Reinit To Default"() -> ()  [unwired: 3 in, 3 out]
          }
        }
        n288 = case shown="True" "btn clr niScope" {
          frame False {
          }
          frame True {
            # "clear niScope chn list"
            n289 = invoke on="niSc channels" class="Arr" method="Reinit To Default"() -> ()  [unwired: 3 in, 3 out]
          }
        }
        n290 = case shown="True" "btn clr cdaq" {
          frame False {
          }
          frame True {
            # "clear cDAQ chn list"
            n291 = invoke on="cDAQ chns" class="Arr" method="Reinit To Default"() -> ()  [unwired: 3 in, 3 out]
          }
        }
      }
      event "btn rem last dmm", "btn rem last niScope", "btn rem last cdaq": Value Change {
        # "Remove last item from channel list"
        n292 = event-data() -> ()  [unwired: 1 in, 6 out]
        n293 = case shown="True" "btn rem last dmm" {
          frame False {
          }
          frame True {
            n294 = local read "DMM Channels"() -> (w387:T15[])
            n295 = Array Size(array=w387) -> (size(s)=w386:i32)
            n296 = Decrement(x=w386) -> (x-1=w385:i32)
            n297 = Array Subset(array=w387, length=w385) -> (w384:T15[])  [unwired: 1 in]
            n298 = local write "DMM Channels"(w384) -> ()
          }
        }
        n299 = case shown="True" "btn rem last niScope" {
          frame False {
          }
          frame True {
            n300 = local read "niSc channels"() -> (w379:T4[])
            n301 = Array Size(array=w379) -> (size(s)=w378:i32)
            n302 = Decrement(x=w378) -> (x-1=w377:i32)
            n303 = Array Subset(array=w379, length=w377) -> (w376:T4[])  [unwired: 1 in]
            n304 = local write "niSc channels"(w376) -> ()
          }
        }
        n305 = case shown="True" "btn rem last cdaq" {
          frame False {
          }
          frame True {
            n306 = local read "cDAQ chns"() -> (w383:T78[])
            n307 = Array Size(array=w383) -> (size(s)=w382:i32)
            n308 = Decrement(x=w382) -> (x-1=w381:i32)
            n309 = Array Subset(array=w383, length=w381) -> (w380:T78[])  [unwired: 1 in]
            n310 = local write "cDAQ chns"(w380) -> ()
          }
        }
      }
      event "btn dmm calstr": Value Change {
        # "run DMM CALSTR command"
        n311 = event-data() -> ()  [unwired: 1 in, 6 out]
        n312 = call "3458A CALSTR Panel.vi"() -> ()  [unwired: 11 in, 1 out]
      }
      event "dmm aper rules": Shortcut Menu Selection (User) {
        # "DMM aperture rules pop-up"
        n313 = event-data() -> ("ItemTag"=w388:string)  [unwired: 1 in, 7 out]
        n314 = case shown="\"DMM_POP_DEF_4AP\"" w388 {
          frame Default {
          }
          frame "DMM_POP_DEF_4AP" {
            n315 = local write "dmm aper rules"(string[][] [["1001", "950u"], ["5701", "150u"], ["16001", "50u"], ["100001", "1.4u"]]) -> ()
          }
          frame "DMM_POP_DEF_3AP" {
            n316 = local write "dmm aper rules"(string[][] [["5701", "150u"], ["16001", "50u"], ["100001", "1.4u"]]) -> ()
          }
        }
      }
      event "btn dsdll enum": Value Change {
        # "Digitizer type changed"
        n317 = event-data() -> ()  [unwired: 1 in, 6 out]
        n318 = local read "adc session out"() -> (w398:T2)
        n319 = local read "Digitizer type"() -> (w396:T57)
        n320 = Not Equal?(x=w396, y=ADC_Type."cDAQ ADC") -> (x != y?=w394:bool)
        n321 = Bundle By Name(cluster=w398, "type"=w396) -> (w393:T2)
        n322 = case shown="True" w394 {
          tunnel: w393 -> [w400 w404]
          tunnel: [w400 w403] -> w392
          tunnel: [_ w401] -> w391
          frame False {
          }
          frame True {
            # "kill cDAQ process if running"
            n323 = call "ADC Deactivate Digitizer.vi"("adc session in"=w404) -> ("error out"=w402:errorcluster, "adc session out"=w403:T2)  [unwired: 9 in]
            n324 = call <vilib>:"Clear Errors.vi"("error in (no error)"=w402) -> ("error out"=w401:errorcluster)  [unwired: 5 in, 1 out]
          }
        }
        n325 = control-ref of="dsdll capt devs"() -> (w399:refnum<vi>)
        n326 = call "ADC Enumerate Devices.vi"("capture devices ring ref"=w399, "error in"=w391, "adc session in"=w392) -> ("error out"=w397:errorcluster)  [unwired: 7 in, 1 out]
        n327 = call <vilib>:"Clear Errors.vi"("error in (no error)"=w397) -> ()  [unwired: 5 in, 2 out]
      }
      event "btn sim clr": Value Change {
        # "clear simulated ADC list"
        n328 = event-data() -> ()  [unwired: 1 in, 6 out]
        n329 = invoke on="simadc chn cfg" class="Arr" method="Reinit To Default"() -> ()  [unwired: 3 in, 3 out]
      }
      event "simadc chn cfg": Value Change {
        # "value changed in the sim ADC setup"
        n330 = event-data() -> ()  [unwired: 1 in, 6 out]
        n331 = local read "simadc chn cfg"() -> (w409:T59[])
        n332 = Bundle By Name(cluster=T58 {"channels"=[], "range [V]"=0.0, "Ts step [s]"=0.0, "time [s]"=0.0, "fs [Hz]"=0.0, "count"=0, "smpl offset"=0, "set count"=0, "bit res"=0} ("Cluster"), "channels"=w409) -> (w408:T58)
        n333 = call "SimAdc Clear Channels.ctl"("simadc in"=w408) -> ("error out"=w407:errorcluster, "simadc out"=w406:T58)  [unwired: 9 in]
        n334 = Unbundle By Name(w406) -> ("channels"=w405:T59[])
        n335 = call <vilib>:"Clear Errors.vi"("error in (no error)"=w407) -> ()  [unwired: 5 in, 2 out]
        n336 = local write "simadc chn cfg"(w405) -> ()
      }
      event "niSc channels", "DMM Channels", "keDSO channels", "cDAQ chns": Value Change {
        # "channels list change"
        n337 = event-data() -> ()  [unwired: 1 in, 6 out]
        n338 = local read "keDSO channels"() -> (w418:T73[])
        n339 = local read "DMM Channels"() -> (w419:T15[])
        n340 = local read "niSc channels"() -> (w426:T4[])
        n341 = local read "cDAQ chns"() -> (w411:T78[])
        n342 = for {
          tunnel: w419 -> [w531] mode=indexing
          tunnel: [w531] -> w420 mode=indexing if=w529
          n343 = Unbundle By Name(w531) -> ("btn clr"=w530:bool)
          n344 = Not(x=w530) -> (.not. x?=w529:bool)
        }
        n345 = for {
          tunnel: w426 -> [w566] mode=indexing
          tunnel: [w566] -> w425 mode=indexing if=w564
          n346 = Unbundle By Name(w566) -> ("btn clr"=w565:bool)
          n347 = Not(x=w565) -> (.not. x?=w564:bool)
        }
        n348 = for {
          tunnel: w418 -> [w496] mode=indexing
          tunnel: [w496] -> w417 mode=indexing if=w494
          n349 = Unbundle By Name(w496) -> ("btn clr"=w495:bool)
          n350 = Not(x=w495) -> (.not. x?=w494:bool)
        }
        n351 = for {
          tunnel: w411 -> [w461] mode=indexing
          tunnel: [w461] -> w412 mode=indexing if=w459
          n352 = Unbundle By Name(w461) -> ("btn clr"=w460:bool)
          n353 = Not(x=w460) -> (.not. x?=w459:bool)
        }
        n354 = for {
          N -> [w502]
          tunnel: w420 -> [w507] mode=indexing
          shift-right: [w500] -> w421
          shift-left: w420 -> [w506]
          i -> [w503]
          n355 = Unbundle By Name(w507) -> ("btn up"=w508:bool, "btn down"=w504:bool)
          n356 = Decrement(x=w502) -> (x-1=w501:i32)
          n357 = case shown="True" w508 {
            tunnel: w506 -> [w519 w528]
            tunnel: w503 -> [_ w526]
            tunnel: [w519 w521] -> w505
            frame False {
            }
            frame True {
              n358 = Decrement(x=w526) -> (x-1=w520:i32)
              n359 = Delete From Array(array=w528, length=1, index=w526) -> (deleted portion=w522:T15[], array with subset deleted=w523:T15[])
              n360 = Max & Min(x=w520, y=0) -> (max(x,y)=w524:i32)  [unwired: 1 out]
              n361 = Insert Into Array(array=w523, index=w524, new element=w522) -> (w521:T15[])
            }
          }
          n362 = case shown="True" w504 {
            tunnel: w505 -> [w509 w518]
            tunnel: w503 -> [_ w516]
            tunnel: [w509 w513] -> w500
            tunnel: w501 -> [_ w512]
            frame False {
            }
            frame True {
              n363 = Increment(x=w516) -> (x+1=w510:i32)
              n364 = Delete From Array(array=w518, length=1, index=w516) -> (deleted portion=w514:T15[], array with subset deleted=w515:T15[])
              n365 = Max & Min(x=w510, y=w512) -> (min(x,y)=w511:i32)  [unwired: 1 out]
              n366 = Insert Into Array(array=w515, index=w511, new element=w514) -> (w513:T15[])
            }
          }
        }
        n367 = for {
          N -> [w537]
          tunnel: w425 -> [w542] mode=indexing
          shift-right: [w535] -> w424
          shift-left: w425 -> [w541]
          i -> [w538]
          n368 = Unbundle By Name(w542) -> ("btn up"=w543:bool, "btn down"=w539:bool)
          n369 = Decrement(x=w537) -> (x-1=w536:i32)
          n370 = case shown="True" w543 {
            tunnel: w541 -> [w554 w563]
            tunnel: w538 -> [_ w561]
            tunnel: [w554 w556] -> w540
            frame False {
            }
            frame True {
              n371 = Decrement(x=w561) -> (x-1=w555:i32)
              n372 = Delete From Array(array=w563, length=1, index=w561) -> (deleted portion=w557:T4[], array with subset deleted=w558:T4[])
              n373 = Max & Min(x=w555, y=0) -> (max(x,y)=w559:i32)  [unwired: 1 out]
              n374 = Insert Into Array(array=w558, index=w559, new element=w557) -> (w556:T4[])
            }
          }
          n375 = case shown="True" w539 {
            tunnel: w540 -> [w544 w553]
            tunnel: w538 -> [_ w551]
            tunnel: [w544 w548] -> w535
            tunnel: w536 -> [_ w547]
            frame False {
            }
            frame True {
              n376 = Increment(x=w551) -> (x+1=w545:i32)
              n377 = Delete From Array(array=w553, length=1, index=w551) -> (deleted portion=w549:T4[], array with subset deleted=w550:T4[])
              n378 = Max & Min(x=w545, y=w547) -> (min(x,y)=w546:i32)  [unwired: 1 out]
              n379 = Insert Into Array(array=w550, index=w546, new element=w549) -> (w548:T4[])
            }
          }
        }
        n380 = for {
          N -> [w467]
          tunnel: w417 -> [w472] mode=indexing
          shift-right: [w465] -> w416
          shift-left: w417 -> [w471]
          i -> [w468]
          n381 = Unbundle By Name(w472) -> ("btn up"=w473:bool, "btn down"=w469:bool)
          n382 = Decrement(x=w467) -> (x-1=w466:i32)
          n383 = case shown="True" w473 {
            tunnel: w471 -> [w484 w493]
            tunnel: w468 -> [_ w491]
            tunnel: [w484 w486] -> w470
            frame False {
            }
            frame True {
              n384 = Decrement(x=w491) -> (x-1=w485:i32)
              n385 = Delete From Array(array=w493, length=1, index=w491) -> (deleted portion=w487:T73[], array with subset deleted=w488:T73[])
              n386 = Max & Min(x=w485, y=0) -> (max(x,y)=w489:i32)  [unwired: 1 out]
              n387 = Insert Into Array(array=w488, index=w489, new element=w487) -> (w486:T73[])
            }
          }
          n388 = case shown="True" w469 {
            tunnel: w470 -> [w474 w483]
            tunnel: w468 -> [_ w481]
            tunnel: [w474 w478] -> w465
            tunnel: w466 -> [_ w477]
            frame False {
            }
            frame True {
              n389 = Increment(x=w481) -> (x+1=w475:i32)
              n390 = Delete From Array(array=w483, length=1, index=w481) -> (deleted portion=w479:T73[], array with subset deleted=w480:T73[])
              n391 = Max & Min(x=w475, y=w477) -> (min(x,y)=w476:i32)  [unwired: 1 out]
              n392 = Insert Into Array(array=w480, index=w476, new element=w479) -> (w478:T73[])
            }
          }
        }
        n393 = for {
          N -> [w432]
          tunnel: w412 -> [w437] mode=indexing
          shift-right: [w430] -> w413
          shift-left: w412 -> [w436]
          i -> [w433]
          n394 = Unbundle By Name(w437) -> ("btn up"=w438:bool, "btn down"=w434:bool)
          n395 = Decrement(x=w432) -> (x-1=w431:i32)
          n396 = case shown="True" w438 {
            tunnel: w436 -> [w449 w458]
            tunnel: w433 -> [_ w456]
            tunnel: [w449 w451] -> w435
            frame False {
            }
            frame True {
              n397 = Decrement(x=w456) -> (x-1=w450:i32)
              n398 = Delete From Array(array=w458, length=1, index=w456) -> (deleted portion=w452:T78[], array with subset deleted=w453:T78[])
              n399 = Max & Min(x=w450, y=0) -> (max(x,y)=w454:i32)  [unwired: 1 out]
              n400 = Insert Into Array(array=w453, index=w454, new element=w452) -> (w451:T78[])
            }
          }
          n401 = case shown="True" w434 {
            tunnel: w435 -> [w439 w448]
            tunnel: w433 -> [_ w446]
            tunnel: [w439 w443] -> w430
            tunnel: w431 -> [_ w442]
            frame False {
            }
            frame True {
              n402 = Increment(x=w446) -> (x+1=w440:i32)
              n403 = Delete From Array(array=w448, length=1, index=w446) -> (deleted portion=w444:T78[], array with subset deleted=w445:T78[])
              n404 = Max & Min(x=w440, y=w442) -> (min(x,y)=w441:i32)  [unwired: 1 out]
              n405 = Insert Into Array(array=w445, index=w441, new element=w444) -> (w443:T78[])
            }
          }
        }
        n406 = for {
          tunnel: w421 -> [w499] mode=indexing
          tunnel: [w497] -> w422 mode=indexing
          w498 = FALSE ("btn up")
          n407 = Bundle By Name(cluster=w499, "btn up"=w498, "btn down"=w498) -> (w497:T15)
        }
        n408 = for {
          tunnel: w424 -> [w534] mode=indexing
          tunnel: [w532] -> w423 mode=indexing
          w533 = FALSE ("btn up")
          n409 = Bundle By Name(cluster=w534, "btn up"=w533, "btn down"=w533) -> (w532:T4)
        }
        n410 = for {
          tunnel: w416 -> [w464] mode=indexing
          tunnel: [w462] -> w415 mode=indexing
          w463 = FALSE ("btn up")
          n411 = Bundle By Name(cluster=w464, "btn up"=w463, "btn down"=w463) -> (w462:T73)
        }
        n412 = for {
          tunnel: w413 -> [w429] mode=indexing
          tunnel: [w427] -> w414 mode=indexing
          w428 = FALSE ("btn up")
          n413 = Bundle By Name(cluster=w429, "btn up"=w428, "btn down"=w428) -> (w427:T78)
        }
        n414 = local write "keDSO channels"(w415) -> ()
        n415 = local write "DMM Channels"(w422) -> ()
        n416 = local write "niSc channels"(w423) -> ()
        n417 = local write "cDAQ chns"(w414) -> ()
      }
      event "btn cfg AWG": Value Change {
        # "AWG clock source config"
        n418 = event-data() -> ()  [unwired: 1 in, 6 out]
        n419 = local read "AWG VISA"() -> (w570:refnum<visa-resource-name>)
        n420 = local read "AWG type"() -> (w567:T19)
        n421 = local read "adc session out"() -> (w571:T2)
        n422 = Bundle By Name(cluster=w571, "3458A.awg unit.type"=w567, "3458A.awg unit.VISA"=w570) -> (w572:T2)
        n423 = Unbundle By Name(w572) -> ("3458A.awg unit"=w575:T18)
        n424 = call "AWG Config Panel.vi"("awg session"=w575) -> ("error out"=w573:errorcluster, "awg session out"=w574:T18)  [unwired: 9 in]
        n425 = Bundle By Name(cluster=w572, "3458A.awg unit"=w574) -> (w569:T2)
        n426 = call <vilib>:"Clear Errors.vi"("error in (no error)"=w573) -> ()  [unwired: 5 in, 2 out]
        n427 = Unbundle By Name(w569) -> ("3458A.awg unit.VISA"=w568:refnum<visa-resource-name>)
        n428 = local write "adc session out"(w569) -> ()
        n429 = local write "AWG VISA"(w568) -> ()
      }
      event "help": Value Change {
        n430 = event-data() -> ()  [unwired: 1 in, 6 out]
        n431 = Control Help Window(1:"help") -> ()  [unwired: 1 in]
      }
    }
    n432 = call <vilib>:"Clear Errors.vi"("error in (no error)"=w97) -> ()  [unwired: 5 in, 2 out]
  }
  n433 = for {
    tunnel: [w578] -> w29 mode=indexing
    tunnel: w28 -> [w577] mode=indexing
    n434 = for {
      tunnel: [w580] -> w578 mode=indexing
      tunnel: w577 -> [w579] mode=indexing
      n435 = Format Into String(format string="%#_4p" ("delimiter (Tab)"), w579) -> (resulting string=w580:string)  [unwired: 2 in, 1 out]
    }
  }
  n436 = local write "dmm aper rules"(w29) -> ()
  n437 = flat-sequence {
    tunnel: w74 -> [_]
    tunnel: w40 -> [w587]
    tunnel: w39 -> [w586]
    frame #0 {
      w588 = SGUI_Assign_References_Mode."Release ID" ("register mode (overwrite)")
      # "unregister controls\nof this panel"
      # "unregister controls of this panel"
      # "on panel close action"
      n438 = local read "adc session out"() -> (w584:T2)
      n439 = call "ADC Reset Idle Timer.vi"("set busy (False)"=FALSE, "adc session in"=w584) -> ("error out"=w585:errorcluster, "adc session out"=w583:T2)  [unwired: 8 in]
      n440 = local write "adc session out"(w583) -> ()
      n441 = call "SGUI Register Controls.vi"("error in"=w585, "register mode (overwrite)"=w588, "controls ID (empty)"=w587) -> ("error out"=w590:errorcluster)  [unwired: 14 in, 2 out]
      n442 = call "SGUI Register Controls Groups.vi"("error in"=w590, "register mode (overwrite)"=w588, "controls ID (empty)"=w586) -> ("error out"=w589:errorcluster)  [unwired: 15 in, 1 out]
      n443 = call <vilib>:"Clear Errors.vi"("error in (no error)"=w589) -> ()  [unwired: 5 in, 2 out]
    }
  }
  "error out" <- "error in"
  "adcstr" <- "" ("adcstr")
